vi "运维调试_总磷总氮.vi"() -> ()   [LabVIEW 2016, in "斯坦道总磷总氮.lvlib"]
uses:
  <vilib>/Utility/miscctls.llb/LVPointTypeDef.ctl
  <vilib>/Utility/config.llb/NI_LVConfig.lvlib
  <vilib>/ptbypt/NI_PtbyPt.lvlib
panel:
  out "固件版本号":string
  in  "定时设置":cluster{"启动":bool, "控制命令":T1, "测量参数":T2}(xcontrol)
  out "模块版本号":string
  out "温度2":sgl
  out "温度1":sgl
  out "ADC":sgl
  out "F3":sgl format="%#.6f"
  out "F2":sgl format="%#.6f"
  out "F1":sgl format="%#.6f"
  out "F0":sgl format="%#.6f"
  out "运行状态":T3 {"数据时间:" format="%<%y/%m/%d %H:%M:%S>T"; "仪器时间:" format="%<%y/%m/%d %H:%M:%S>T"}
  in  "单选按钮":enum32{"选项卡 1", "选项卡 2"}(radio)
  in  "总磷参数设置":bool
  in  "总氮参数设置":bool
  out "二级权限":bool
  out "一级权限":bool
  out "输入密码":u32
  out "布尔":bool
  in  "流程固件":bool
  in  "量程参数读取":T4
  in  "模块启用":bool
  in  "串口设置":bool
  in  "公式一键写入":bool
  in  "流程路径":path=path "C:/Users/Hsiao/Documents/斯坦道流程文件/流程.xml"
  in  "曲线模型":cluster{"X^2":dbl, "X":dbl, "B":dbl, "r^2":dbl}(xcontrol)
  out "字符串 2":string
  in  "质控参数设置":bool
  in  "总氮自动测试量程配置":T5
  in  "总磷自动测试量程配置":T5
  in  "数组":string[](array[string])
  in  "量程切换阈值写入":bool
  in  "量程切换阈值读取":bool
  in  "参数下拉列表":enum16{"总磷", "总氮"}(ring)
  in  "量程下拉列表":enum16{"低量程", "高量程"}(ring)
  in  "测量模式下拉列表":enum16{"水样测量", "零点核查", "跨度核查", "标样核查", "加标回收"}(ring)
  in  "公式":cluster{"X^2":dbl, "X":dbl, "b":dbl}
  in  "写公式":bool
  in  "读公式":bool
  in  "返回":bool
  in  "参数设置":bool
  out "集成报警信息":string
  in  "停止":bool
  in  "手动启动":bool
  in  "单步测试":bool
  out "多列列表框":i32(listbox)
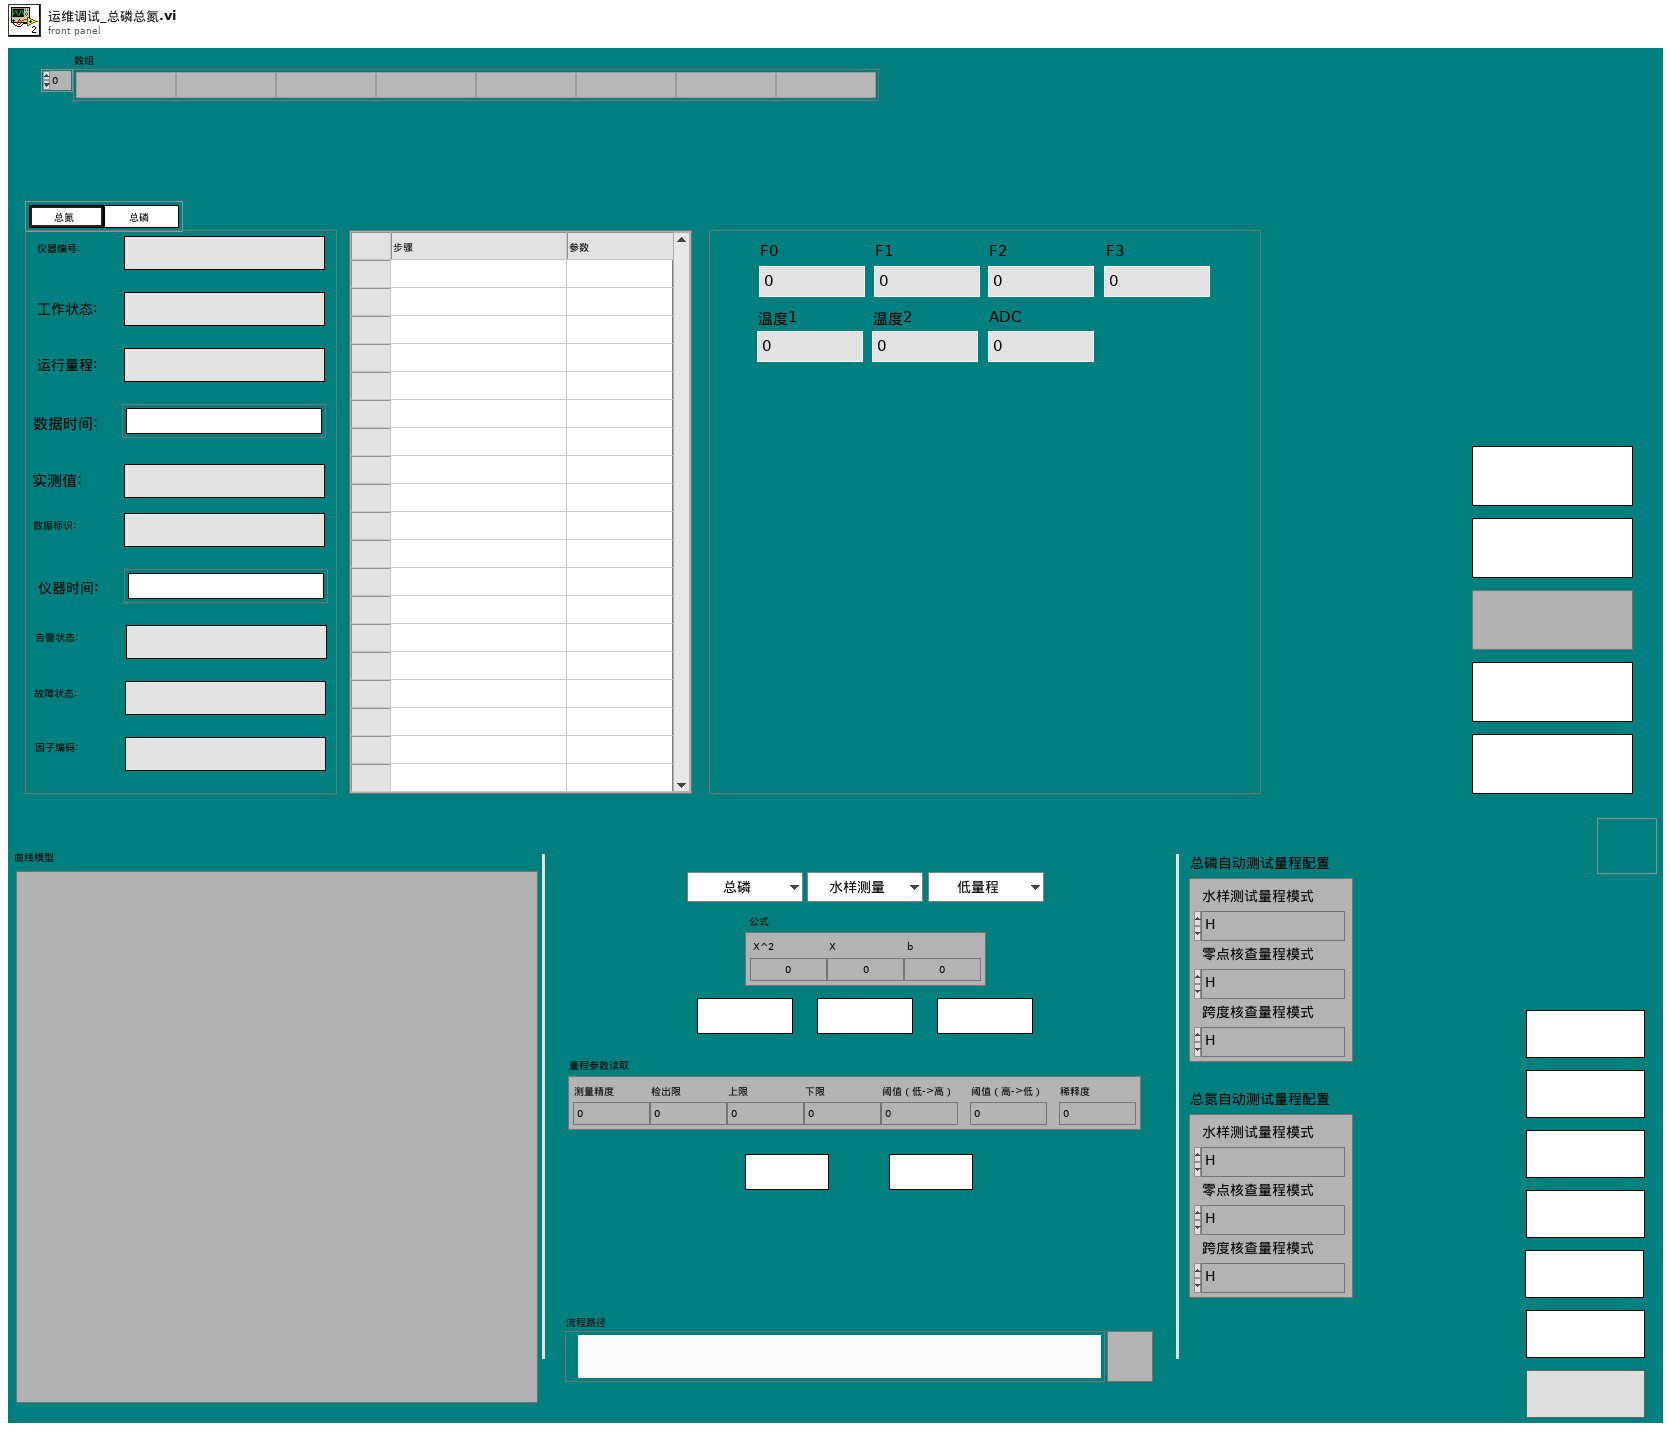
[diagram p1: front panel]
types:
  T1 = typedef "定时设置.xctl/国标控制命令.ctl" = enum16{"启动测量", "标样核查", "零点核查", "跨度核查", "空白测试", "平行样测试", "加标回收", "空白校准", "标样校准", "初始化（清洗）", "停止测试", "仪器重启", "校时", "模式设置", "测量间隔设置"}
  T2 = typedef "定时设置.xctl/测量参数.ctl" = u16
  T3 = cluster{"仪器编号:":string, "工作状态:":string, "运行量程: ":string, "数据时间:":timestamp, "实测值:":string, "数据标识: ":string, "仪器时间:":timestamp, "告警状态: ":string, "故障状态:  ":string, "因子编码:":string}
  T4 = cluster{"测量精度":dbl, "检出限":dbl, "上限":dbl, "下限":dbl, "阈值（低->高）":dbl, "阈值（高->低）":dbl, "稀释度":dbl}
  T5 = cluster{"水样测试量程模式":enum16{"H", "L", "AUTO"}, "空白核查量程模式":enum16{"H", "L", "AUTO"}, "跨度核查量程模式":enum16{"H", "L", "AUTO"}}
  T6 = cluster{"时间源选择":enum16{"系统时间源", "仪器时间源"}, "外部时间源":timestamp}
  T7 = cluster{"系统时间":timestamp, "工作状态":enum16{"空闲", "水样测试", "标样核查", "零点核查", "跨度核查", "空白测试", "平行样测试", "加标回收", "空白校准", "标样校准", "初始化（清洗）"}, "测量模式":enum16{"待机", "连续模式", "周期模式", "定点模式", "受控模式", "手动模式"}, "告警代码":u16, "故障代码":u16, "日志代码":u16, "软件版本":u16, "F0":sgl, "F1":sgl, "F2":sgl, "F3":sgl, "T":sgl, "H":sgl, "id":u16, "flowid":u16, "量程":u16, "总磷控温温度1":sgl, "营养盐控温温度2":sgl, "ADC":sgl}
  T8 = enum16{"空闲", "水样测试", "标样核查", "零点核查", "跨度核查", "空白测试", "平行样测试", "加标回收", "空白校准", "标样校准", "初始化（清洗）"}
  T9 = enum32{"Bad", "Idle", "Run top level", "Running"}
  T10 = typedef "定时设置.xctl/周期模式设置.ctl" = enum16{"不启用", "定点模式", "间隔模式"}
  T11 = typedef "定时设置.xctl/定点周期设置.ctl" = cluster{"启动命令":T12, "启动命令 2":T12, "启动命令 3":T12, "启动命令 4":T12, "启动命令 5":T12, "启动命令 6":T12, "启动命令 7":T12, "启动命令 8":T12, "启动命令 9":T12, "启动命令 10":T12, "启动命令 11":T12, "启动命令 12":T12, "启动命令 13":T12, "启动命令 14":T12, "启动命令 15":T12, "启动命令 16":T12, "启动命令 17":T12, "启动命令 18":T12, "启动命令 19":T12, "启动命令 20":T12, "启动命令 21":T12, "启动命令 22":T12, "启动命令 23":T12, "启动命令 24":T12}
  T12 = typedef "定时设置.xctl/启动命令选择.ctl" = u16
  T13 = typedef "定时设置.xctl/间隔启动设置.ctl" = cluster{"启动命令":T12, "启动间隔":dbl, "启动次数":i32}
  T14 = cluster{"周期模式":T10, "定点周期":T11, "间隔启动":T13, "测量参数":T2}
  T15 = typedef "NI_LVConfig.lvlib/Config Data RefNum.ctl" = refnum<k1>
  T16 = typedef "LVPointTypeDef.ctl" = cluster{"Horizontal":i16, "Vertical":i16}
  T17 = cluster{"因子编码":u32, "单位":u16, "标样参考值":sgl, "水样数据时间":timestamp, "水样实测值":sgl, "水样数据标识":string, "标样数据时间":timestamp, "标样实测值":sgl, "标样数据标识":string, "空白数据时间":timestamp, "空白实测值":sgl, "空白数据标识":string, "零点核查数据时间":timestamp, "零点核查实测值":sgl, "零点核查数据标识":string, "跨度核查数据时间":timestamp, "跨度核查实测值":sgl, "跨度核查数据标识":string, "加标回收数据时间":timestamp, "加标回收实测值":sgl, "加标回收数据标识":string, "平行样数据时间":timestamp, "平行样实测值":sgl, "平行样数据标识":string, "F0":sgl, "F1":sgl, "F2":sgl, "F3":sgl, "F4":sgl, "F5":sgl, "F6":sgl, "F7":sgl, "温度":sgl, "湿度":sgl, "X值":sgl, "fidrange":u16}
  T18 = cluster{"Major":u16, "Minor":u16, "Fix":u16, "Build":u16}
  T19 = enum8{"Enabled", "Disabled", "Disabled and Grayed Out"}
  T20 = cluster{"时间标识":timestamp, "设备":string, "日志信息":string, "备注":string}
  T21 = cluster{"参数":string, "报警内容":string, "报警分析":string}
  T22 = cluster{"启动模式":enum16{"跨度核查", "水样测量", "空白核查", "标样核查", "加标回收"}, "启动参数":u16, "量程":enum16{"低量程", "高量程"}}
  T23 = cluster{"时间标识":timestamp, "设备":string, "日志信息":string, "流程参数":string}
  T24 = typedef "LVRowAndColumnUnsignedTypeDef.ctl" = cluster{"Row":u32, "Column":u32}
  T25 = cluster{"参数下拉列表":enum16{"总磷", "总氮"}, "测量模式下拉列表":enum16{"水样测量", "零点核查", "跨度核查", "标样核查", "加标回收"}, "量程下拉列表":enum16{"低量程", "高量程"}}
  T26 = cluster{"站号":u16, "量程切换":enum32{"H", "L", "AUTO"}, "控制命令":enum16{"启动测量", "标样核查", "零点核查", "跨度核查", "空白测试", "平行样测试", "加标回收", "空白校准", "标样校准", "初始化（清洗）", "停止测试", "仪器重启", "校时", "模式设置", "测量间隔设置"}, "模式设置":enum16{"待机", "连续模式", "周期模式", "定点模式", "受控模式", "手动模式"}, "测量间隔":u16}
  T27 = cluster{"总磷跨度值":dbl, "总磷零点标准液浓度":dbl, "总磷跨度标准液浓度":dbl, "总磷标准液标准浓度":dbl, "总氮跨度值":dbl, "总氮零点标准液浓度":dbl, "总氮跨度标准液浓度":dbl, "总氮标准液标准浓度":dbl}
  T28 = cluster{"确定":bool, "总磷跨度值":dbl, "总磷零点标准液浓度":dbl, "总磷跨度标准液浓度":dbl, "总磷标准液标准浓度":dbl, "总氮跨度值":dbl, "总氮零点标准液浓度":dbl, "总氮跨度标准液浓度":dbl, "总氮标准液标准浓度":dbl}
  T29 = cluster{"测量量程":dbl, "测量精度":dbl, "测量间隔":dbl, "消解温度":dbl, "消解时长":dbl, "空白校准时间":timestamp, "曲线截距":dbl, "曲线斜率":dbl, "测量检出限":dbl, "测量信号值":dbl, "线性相关系数":dbl, "二次多项式系数":dbl, "标样校准时间":timestamp, "稀释倍数":dbl, "三项式系数":dbl, "空白标定系数":dbl, "量程系数":dbl, "F0/ORPA":dbl, "F1/ORPB":dbl, "F2/ORPK":dbl, "F3":dbl, "F4":dbl, "F5":dbl, "F6":dbl, "F7":dbl, "X0/滴定数":dbl, "量程":dbl}
  T30 = cluster{"确定":bool, "测量量程":dbl, "测量精度":dbl, "测量间隔":dbl, "消解温度":dbl, "消解时长":dbl, "空白校准时间":timestamp, "曲线截距":dbl, "曲线斜率":dbl, "测量检出限":dbl, "测量信号值":dbl, "线性相关系数":dbl, "二次多项式系数":dbl, "标样校准时间":timestamp, "稀释倍数":dbl, "三项式系数":dbl, "空白标定系数":dbl, "量程系数":dbl, "F0/ORPA":dbl, "F1/ORPB":dbl, "F2/ORPK":dbl, "F3":dbl, "F4":dbl, "F5":dbl, "F6":dbl, "F7":dbl, "X0/滴定数":dbl, "量程":dbl}
  T31 = cluster{"测量精度":u16, "检出限":dbl, "上限":dbl, "下限":dbl, "阈值（低->高）":dbl, "阈值（高->低）":dbl, "稀释度":dbl}
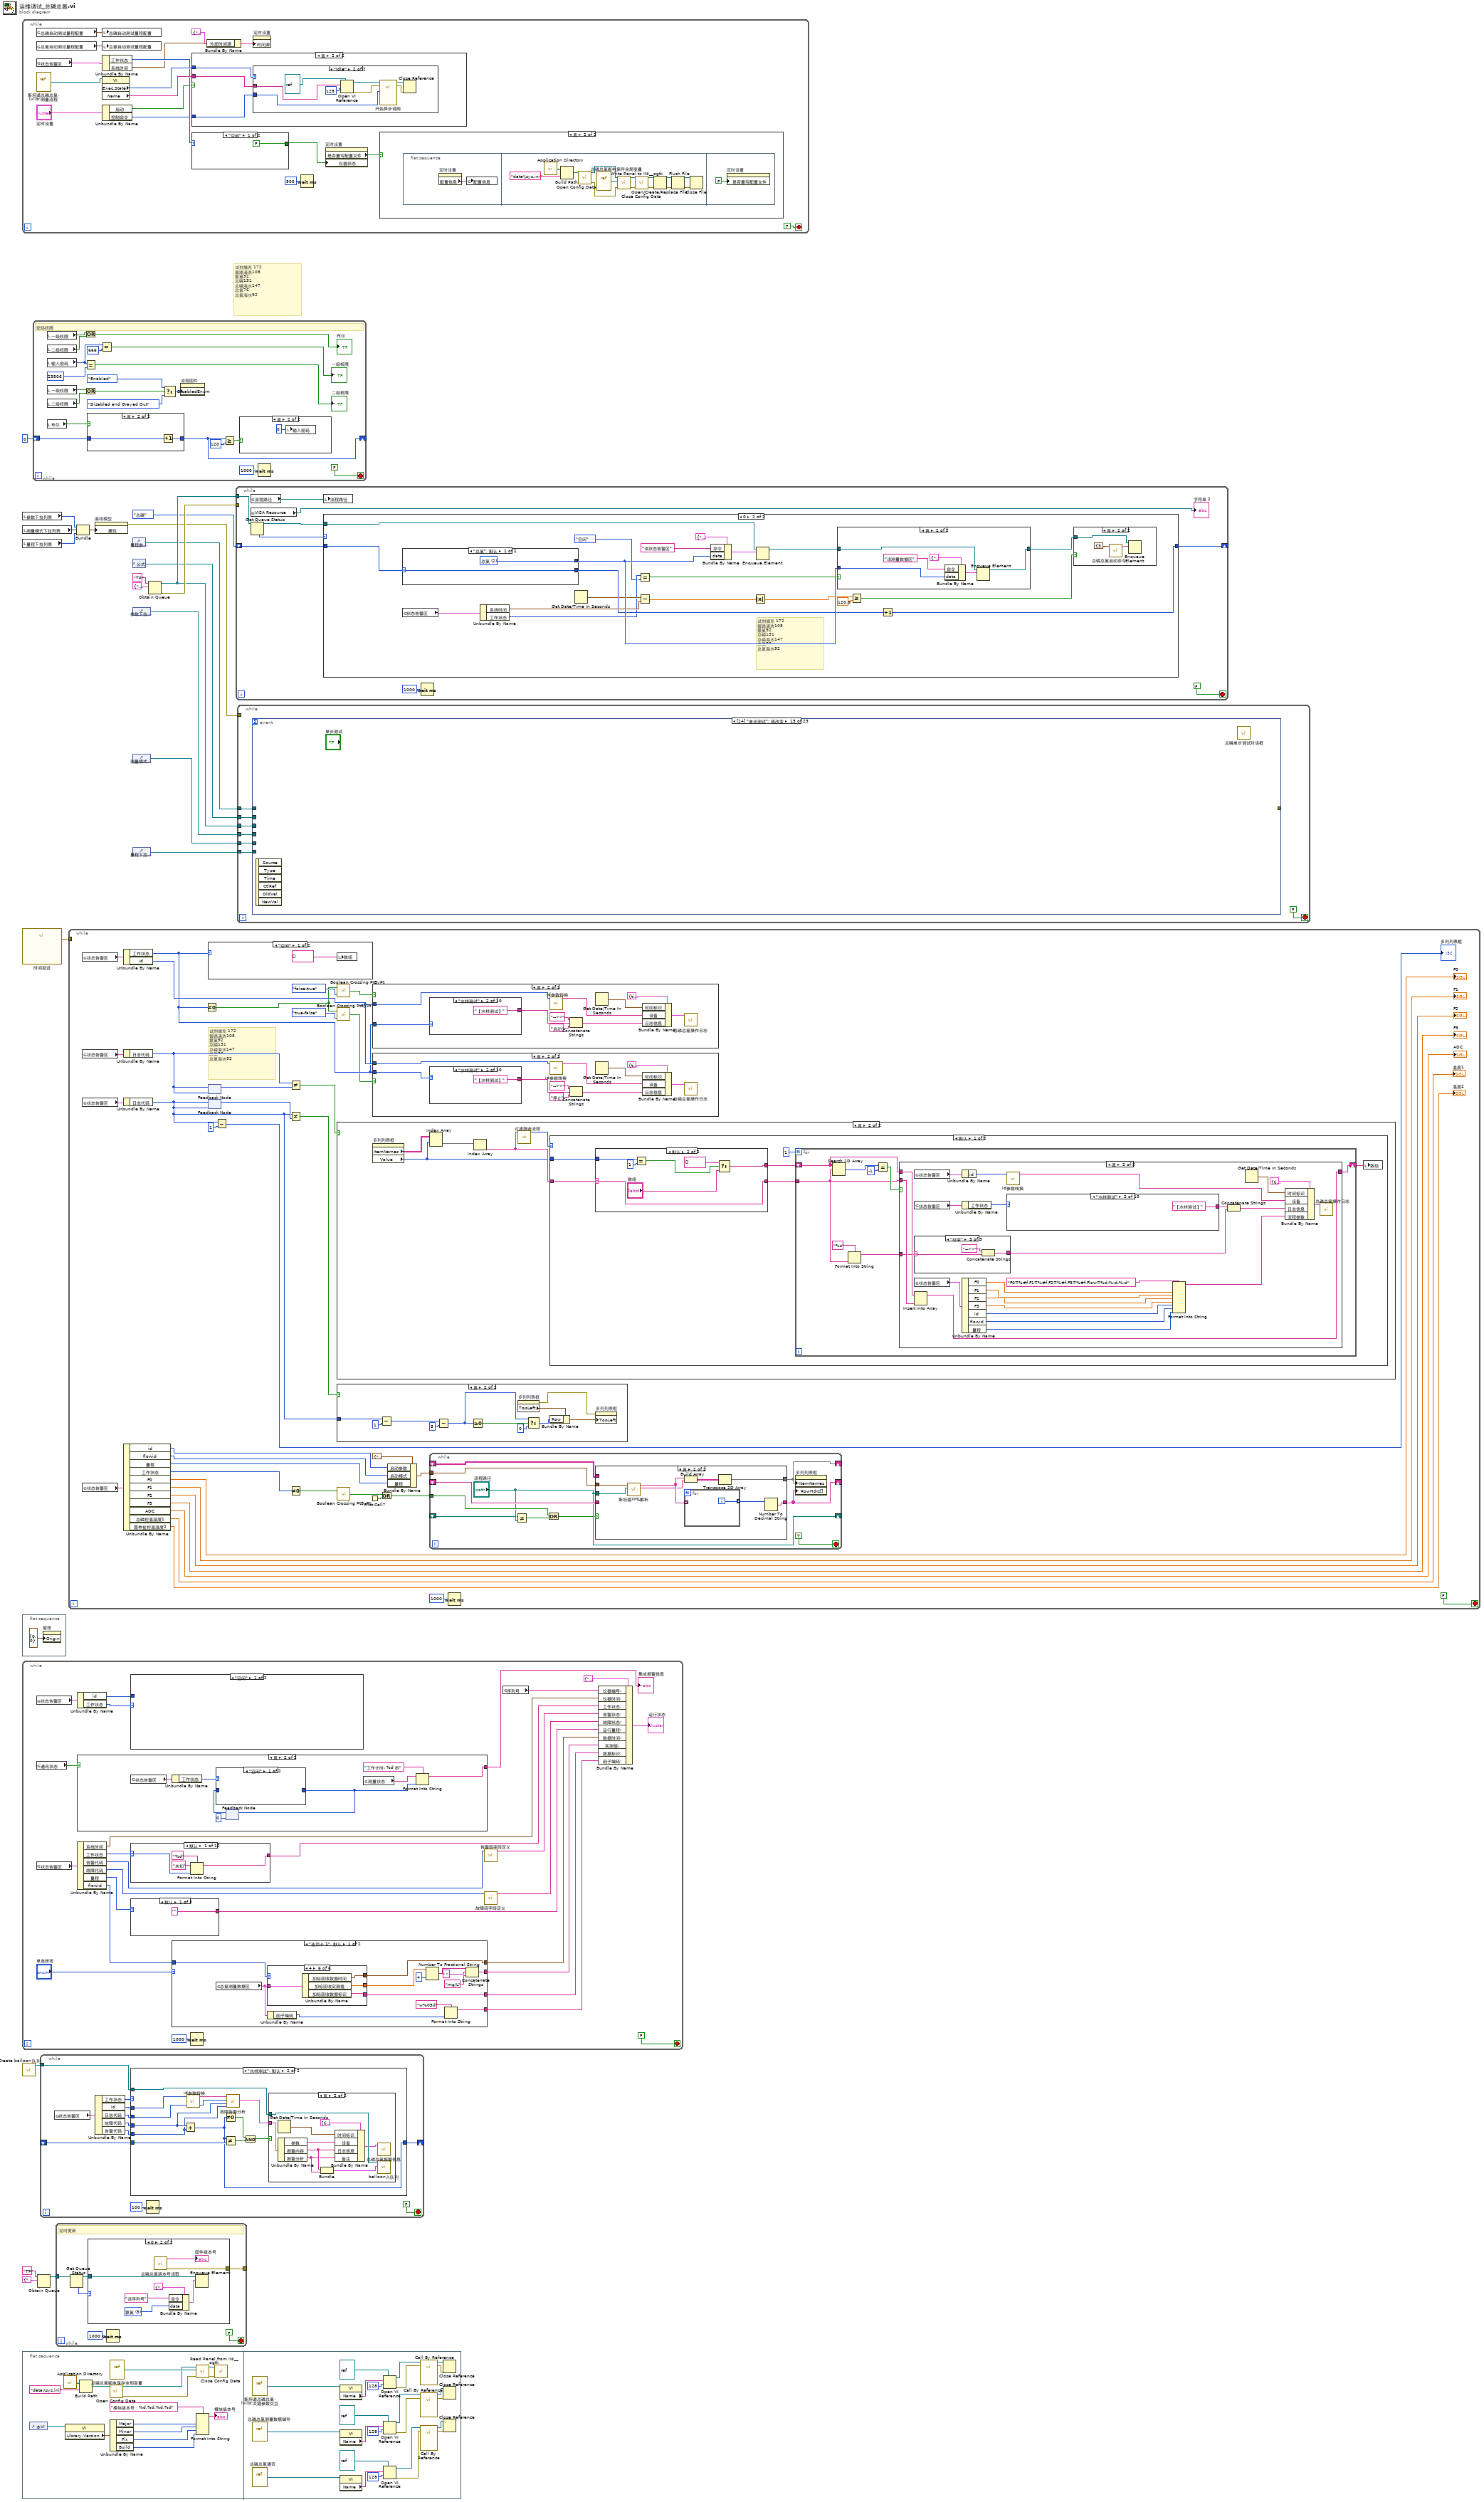
[diagram p0: block diagram]
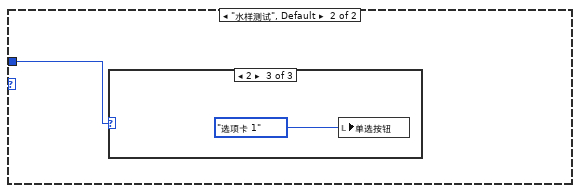
[diagram p7: hidden frame]
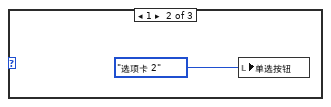
[diagram p9: hidden frame]
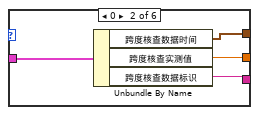
[diagram p11: hidden frame]
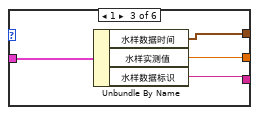
[diagram p12: hidden frame]
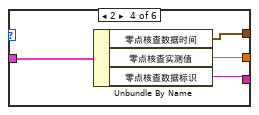
[diagram p13: hidden frame]
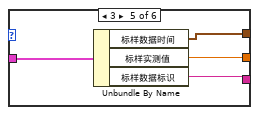
[diagram p14: hidden frame]
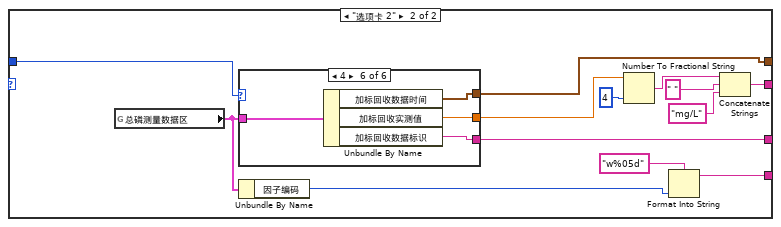
[diagram p15: hidden frame]
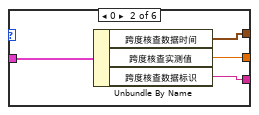
[diagram p17: hidden frame]
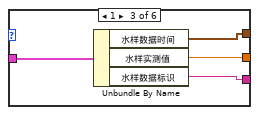
[diagram p18: hidden frame]
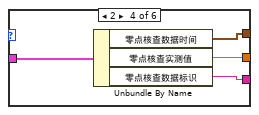
[diagram p19: hidden frame]
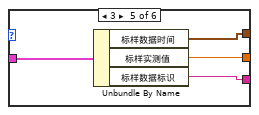
[diagram p20: hidden frame]
diagram:
  # "试剂填充 172 \n管路清洗108\n氨氮92\n总磷131\n总磷海水147\n总氮76\n总氮海水92"
  n1 = while {
    stop <- FALSE stop-if-true
    n2 = global read "总磷总氮断电保存全局变量.vi" "总磷自动测试量程配置"() -> (w35:T5)
    n3 = global read "总磷总氮断电保存全局变量.vi" "总氮自动测试量程配置"() -> (w36:T5)
    n4 = global read "VAR总磷总氮全局变量.vi" "状态告警区"() -> (w31:T7)
    n5 = vi-ref "斯坦道总磷总氮.lvlib:测量流程.vi"() -> (w34:refnum<vi>)
    n6 = local write "总磷自动测试量程配置"(w35) -> ()
    n7 = local write "总氮自动测试量程配置"(w36) -> ()
    n8 = Unbundle By Name(w31) -> ("工作状态"=w30:T8, "系统时间"=w22:timestamp)
    n9 = property class="VI"(reference=w34) -> ("Exec.State"=w33:T9, "Name"=w32:string)  [unwired: 1 in, 2 out]
    n10 = Unbundle By Name("定时设置") -> ("启动"=w26:bool, "控制命令"=w25:T1)
    n11 = case shown="真" w26 {
      tunnel: w32 -> [_ w60]
      tunnel: w25 -> [_ w59]
      tunnel: w33 -> [_ w58]
      frame False {
      }
      frame True {
        n12 = case shown="\"Idle\"" w58 {
          tunnel: w60 -> [_ w64]
          tunnel: w59 -> [_ w61]
          frame "Bad", Default {
          }
          frame "Idle" {
            n13 = Open VI Reference(type specifier VI Refnum (for type only)=refnum<vi> refnum, vi path=w64, options=128 ("选项")) -> (vi reference=w65:refnum<vi>, error out=w66:errorcluster)  [unwired: 3 in]
            n14 = call-by-ref "开始异步调用"(reference=w65, error in=w66, "控制命令"=w61) -> (reference out=w67:refnum<vi>, error out=w68:errorcluster)  [unwired: 11 in]
            n15 = Close Reference(reference=w67, error in (no error)=w68) -> ()  [unwired: 1 out]
          }
        }
      }
    }
    n16 = case shown="\"空闲\"" w30 {
      tunnel: [FALSE TRUE] -> w29
      frame "空闲" {
      }
      frame "水样测试", Default {
      }
    }
    n17 = Bundle By Name(cluster=T6 {"时间源选择"=enum."仪器时间源", "外部时间源"=timestamp(0 s since 1904-01-01)} ("时间源"), "外部时间源"=w22) -> (w23:T6)
    n18 = property on="定时设置" class="定时设置 (严格)"("时间源"=w23) -> ()  [unwired: 2 in, 2 out]
    n19 = Wait (ms)(milliseconds to wait=u32 500 ("等待时间（毫秒）")) -> ()  [unwired: 1 out]
    n20 = property on="定时设置" class="定时设置 (严格)"("仪器状态"=w29) -> ("是否重写配置文件"=w28:bool)  [unwired: 2 in, 2 out]
    n21 = case shown="真" w28 {
      frame False {
        n22 = global read "总磷总氮断电保存全局变量.vi" "配置信息"() -> (w39:T14)
        n23 = property on="定时设置" class="定时设置 (严格)"("配置信息"=w39) -> ()  [unwired: 2 in, 2 out]
      }
      frame True {
        n24 = flat-sequence {
          frame #0 {
            n25 = property on="定时设置" class="定时设置 (严格)"() -> ("配置信息"=w40:T14)  [unwired: 2 in, 2 out]
            n26 = global write "总磷总氮断电保存全局变量.vi" "配置信息"(w40) -> ()
          }
          frame #1 {
            n27 = call <vilib>:"Application Directory.vi"() -> ("Application Directory"=w54:path)
            n28 = Build Path(base path=w54, name or relative path="data\\sys.ini" ("名称或相对路径")) -> (appended path=w52:path)
            n29 = call <vilib>:"Open Config Data.vi"("configuration file path"=w52) -> ("error out"=w48:errorcluster, "refnum"=w51:T15)  [unwired: 8 in, 1 out]
            n30 = vi-ref "总磷总氮断电保存全局变量.vi"() -> (w50:refnum<vi>)
            n31 = call <userlib>:"Write Panel to INI__ogtk.vi"("error in (no error)"=w48, "VI ref"=w50, "refnum"=w51) -> ("error out"=w47:errorcluster, "refnum out"=w49:T15)  [unwired: 7 in]
            n32 = call <vilib>:"Close Config Data.vi"("error in (no error)"=w47, "refnum"=w49) -> ("error out"=w42:errorcluster, "file path"=w41:path)  [unwired: 8 in]
            n33 = Open/Create/Replace File(file path (use dialog)=w41, error in=w42) -> (refnum out=w45:refnum<file>, error out=w46:errorcluster)  [unwired: 4 in, 1 out]
            n34 = Flush File(refnum=w45, error in=w46) -> (refnum out=w44:refnum<file>, error out=w43:errorcluster)
            n35 = Close File(refnum=w44, error in=w43) -> ()  [unwired: 2 out]
          }
          frame #2 {
            n36 = property on="定时设置" class="定时设置 (严格)"("是否重写配置文件"=FALSE) -> ()  [unwired: 2 in, 2 out]
          }
        }
      }
    }
  }
  n37 = local read "参数下拉列表"() -> (w5:enum16{"总磷", "总氮"})
  n38 = local read "测量模式下拉列表"() -> (w4:enum16{"水样测量", "零点核查", "跨度核查", "标样核查", "加标回收"})
  n39 = local read "量程下拉列表"() -> (w3:enum16{"低量程", "高量程"})
  n40 = call "时间延迟"() -> ("error out"=w11:errorcluster)  [unwired: 11 in]
  n41 = flat-sequence {
    frame #0 {
      n42 = property on="窗格" class="Pane"("Origin"=T16 {"Horizontal"=0, "Vertical"=0} ("原点")) -> ()  [unwired: 2 in, 2 out]
    }
  }
  n43 = while {
    stop <- FALSE stop-if-true
    n44 = global read "VAR总磷总氮全局变量.vi" "状态告警区"() -> (w76:T7)
    n45 = global read "VAR总磷总氮全局变量.vi" "通讯状态"() -> (w93:bool)
    n46 = global read "VAR总磷总氮全局变量.vi" "状态告警区"() -> (w91:T7)
    n47 = Unbundle By Name(w76) -> ("id"=w75:u16, "工作状态"=w70:T8)
    n48 = case shown="真" w93 {
      tunnel: ["通讯异常" ("集成报警信息") w185] -> w92
      frame False {
      }
      frame True {
        n49 = global read "VAR总磷总氮全局变量.vi" "状态告警区"() -> (w191:T7)
        n50 = Unbundle By Name(w191) -> ("工作状态"=w190:T8)
        n51 = feedback #1(0) -> (w188:i32)
        n52 = case shown="\"空闲\"" w190 {
          tunnel: w188 -> [_ w193]
          tunnel: [_ w192] -> w186
          frame "空闲" {
          }
          frame Default {
            n53 = Increment(x=w193) -> (x+1=w192:i32)
          }
        }
        n54 = feedback-in #1(w186) -> ()
        n55 = global read "VAR总磷总氮全局变量.vi" "测量状态"() -> (w184:string)
        n56 = Format Into String(format string="工作计时: %d 秒" ("格式字符串"), initial string=w184, w186) -> (resulting string=w185:string)  [unwired: 1 in, 1 out]
      }
    }
    "集成报警信息" <- w92
    n57 = Unbundle By Name(w91) -> ("系统时间"=w87:timestamp, "工作状态"=w86:T8, "告警代码"=w74:u16, "故障代码"=w72:u16, "量程"=w84:u16, "flowid"=w81:u16)
    n58 = case shown="\"空闲\"" w70 {
      tunnel: w75 -> [_ w96]
      frame "空闲" {
      }
      frame "水样测试", Default {
        n59 = case shown="2" w96 {
          frame 0, Default {
          }
          frame 1 {
            n60 = local write "单选按钮"(enum32{"选项卡 1", "选项卡 2"}."选项卡 2" ("单选按钮")) -> ()
          }
          frame 2 {
            n61 = local write "单选按钮"(enum32{"选项卡 1", "选项卡 2"}."选项卡 1" ("单选按钮")) -> ()
          }
        }
      }
    }
    n62 = case shown="默认" w86 {
      selector: w86 -> [w168 _ _ _ _ _ _ _ _ _ _ _]
      tunnel: [w169 "空闲" ("工作状态") "水样测量" ("工作状态") "标样核查" ("工作状态") "零点核查" ("工作状态") "跨度核查" ("工作状态") "空白测试" ("工作状态") "平行样测试" ("工作状态") "加标回收" ("工作状态") "空白校准" ("工作状态") "标样校准" ("工作状态") "初始化" ("工作状态")] -> w85
      frame Default {
        n63 = Format Into String(format string="%d" ("格式字符串"), initial string="未知" ("工作状态"), w168) -> (resulting string=w169:string)  [unwired: 1 in, 1 out]
      }
      frame "空闲" {
      }
      frame "水样测试" {
      }
      frame "标样核查" {
      }
      frame "零点核查" {
      }
      frame "跨度核查" {
      }
      frame "空白测试" {
      }
      frame "平行样测试" {
      }
      frame "加标回收" {
      }
      frame "空白校准" {
      }
      frame "标样校准" {
      }
      frame "初始化（清洗）" {
      }
    }
    n64 = case shown="默认" w84 {
      tunnel: ["" ("字符串") "低量程" ("字符串") "高量程" ("字符串")] -> w83
      frame Default {
      }
      frame 0 {
      }
      frame 1 {
      }
    }
    n65 = case shown="\"选项卡 1\", 默认" "单选按钮" {
      tunnel: w81 -> [w103 w136]
      tunnel: [w102 w135] -> w80
      tunnel: [w101 w134] -> w79
      tunnel: [w100 w133] -> w78
      tunnel: [w99 w132] -> w77
      frame "选项卡 1", Default {
        n66 = global read "VAR总磷总氮全局变量.vi" "总氮测量数据区"() -> (w104:T17)
        n67 = case shown="4" w103 {
          tunnel: [_ w115 w119 w123 w127 w131] -> w102
          tunnel: [_ w113 w118 w122 w126 w130] -> w106
          tunnel: [_ w112 w117 w121 w125 w129] -> w100
          tunnel: w104 -> [_ w114 w116 w120 w124 w128]
          frame Default {
          }
          frame 0 {
            n68 = Unbundle By Name(w114) -> ("跨度核查数据时间"=w115:timestamp, "跨度核查实测值"=w113:sgl, "跨度核查数据标识"=w112:string)
          }
          frame 1 {
            n69 = Unbundle By Name(w116) -> ("水样数据时间"=w119:timestamp, "水样实测值"=w118:sgl, "水样数据标识"=w117:string)
          }
          frame 2 {
            n70 = Unbundle By Name(w120) -> ("零点核查数据时间"=w123:timestamp, "零点核查实测值"=w122:sgl, "零点核查数据标识"=w121:string)
          }
          frame 3 {
            n71 = Unbundle By Name(w124) -> ("标样数据时间"=w127:timestamp, "标样实测值"=w126:sgl, "标样数据标识"=w125:string)
          }
          frame 4 {
            n72 = Unbundle By Name(w128) -> ("加标回收数据时间"=w131:timestamp, "加标回收实测值"=w130:sgl, "加标回收数据标识"=w129:string)
          }
        }
        n73 = Unbundle By Name(w104) -> ("因子编码"=w110:u32)
        n74 = Number To Fractional String(number=w106, precision (6)=i16 4 ("精度(6)")) -> (F-format string=w108:string)  [unwired: 2 in]
        n75 = Format Into String(format string="w%05d" ("格式字符串"), w110) -> (resulting string=w99:string)  [unwired: 2 in, 1 out]
        n76 = Concatenate Strings(w108, " " ("字符串"), "mg/L" ("字符串")) -> (w101:string)
      }
      frame "选项卡 2" {
        n77 = global read "VAR总磷总氮全局变量.vi" "总磷测量数据区"() -> (w137:T17)
        n78 = case shown="4" w136 {
          tunnel: [_ w148 w152 w156 w160 w164] -> w135
          tunnel: [_ w146 w151 w155 w159 w163] -> w139
          tunnel: [_ w145 w150 w154 w158 w162] -> w133
          tunnel: w137 -> [_ w147 w149 w153 w157 w161]
          frame Default {
          }
          frame 0 {
            n79 = Unbundle By Name(w147) -> ("跨度核查数据时间"=w148:timestamp, "跨度核查实测值"=w146:sgl, "跨度核查数据标识"=w145:string)
          }
          frame 1 {
            n80 = Unbundle By Name(w149) -> ("水样数据时间"=w152:timestamp, "水样实测值"=w151:sgl, "水样数据标识"=w150:string)
          }
          frame 2 {
            n81 = Unbundle By Name(w153) -> ("零点核查数据时间"=w156:timestamp, "零点核查实测值"=w155:sgl, "零点核查数据标识"=w154:string)
          }
          frame 3 {
            n82 = Unbundle By Name(w157) -> ("标样数据时间"=w160:timestamp, "标样实测值"=w159:sgl, "标样数据标识"=w158:string)
          }
          frame 4 {
            n83 = Unbundle By Name(w161) -> ("加标回收数据时间"=w164:timestamp, "加标回收实测值"=w163:sgl, "加标回收数据标识"=w162:string)
          }
        }
        n84 = Unbundle By Name(w137) -> ("因子编码"=w143:u32)
        n85 = Number To Fractional String(number=w139, precision (6)=i16 4 ("精度(6)")) -> (F-format string=w141:string)  [unwired: 2 in]
        n86 = Format Into String(format string="w%05d" ("格式字符串"), w143) -> (resulting string=w132:string)  [unwired: 2 in, 1 out]
        n87 = Concatenate Strings(w141, " " ("字符串"), "mg/L" ("字符串")) -> (w134:string)
      }
    }
    n88 = Wait (ms)(milliseconds to wait=u32 1000 ("等待时间（毫秒）")) -> ()  [unwired: 1 out]
    n89 = call "告警码字段定义.vi"("告警代码"=w74) -> ("字符串"=w73:string)  [unwired: 8 in, 2 out]
    n90 = call "故障码字段定义.vi"("故障代码"=w72) -> ("字符串"=w71:string)  [unwired: 10 in]
    n91 = global read "VAR总磷总氮全局变量.vi" "序列号"() -> (w88:string)
    n92 = Bundle By Name(cluster=T3 {"仪器编号:"="", "工作状态:"="", "运行量程: "="", "数据时间:"=timestamp(0 s since 1904-01-01), "实测值:"="", "数据标识: "="", "仪器时间:"=timestamp(0 s since 1904-01-01), "告警状态: "="", "故障状态:  "="", "因子编码:"=""} ("运行状态"), "仪器编号:"=w88, "仪器时间:"=w87, "工作状态:"=w85, "告警状态:"=w73, "故障状态:"=w71, "运行量程:"=w83, "数据时间:"=w80, "实测值:"=w79, "数据标识:"=w78, "因子编码:"=w77) -> (→"运行状态":T3)
  }
  n93 = call "Create balloon 队列.vi"() -> ("队列输出"=w1:refnum<queue>)  [unwired: 11 in]
  n94 = flat-sequence {
    frame #0 {
      n95 = control-ref of="本VI"() -> (w201:refnum<vi>)
      n96 = call <vilib>:"Application Directory.vi"() -> ("Application Directory"=w202:path)
      n97 = property class="VI"(reference=w201) -> ("Library.Version"=w200:T18)  [unwired: 1 in, 2 out]
      n98 = Build Path(base path=w202, name or relative path="data\\sys.ini" ("名称或相对路径")) -> (appended path=w204:path)
      n99 = vi-ref "总磷总氮断电保存全局变量.vi"() -> (w206:refnum<vi>)
      n100 = call <vilib>:"Open Config Data.vi"("configuration file path"=w204) -> ("error out"=w208:errorcluster, "refnum"=w205:T15)  [unwired: 8 in, 1 out]
      n101 = Unbundle By Name(w200) -> ("Major"=w198:u16, "Minor"=w197:u16, "Fix"=w196:u16, "Build"=w195:u16)
      n102 = call <userlib>:"Read Panel from INI__ogtk.vi"("error in (no error)"=w208, "VI ref"=w206, "refnum"=w205) -> ("error out"=w209:errorcluster, "refnum out"=w207:T15)  [unwired: 7 in]
      n103 = Format Into String(format string="模块版本号：%d.%d.%d.%d" ("格式字符串"), w198, w197, w196, w195) -> (resulting string=→"模块版本号":string)  [unwired: 2 in, 1 out]
      n104 = call <vilib>:"Close Config Data.vi"("error in (no error)"=w209, "refnum"=w207) -> ()  [unwired: 8 in, 2 out]
    }
    frame #1 {
      n105 = vi-ref "斯坦道总磷总氮.lvlib:关键参数交互.vi"() -> (w217:refnum<vi>)
      n106 = vi-ref "总磷总氮测量数据储存.vi"() -> (w226:refnum<vi>)
      n107 = vi-ref "总磷总氮通讯.vi"() -> (w218:refnum<vi>)
      n108 = property class="VI"(reference=w217) -> ("Name"=w211:string)  [unwired: 1 in, 2 out]
      n109 = property class="VI"(reference=w226) -> ("Name"=w233:string)  [unwired: 1 in, 2 out]
      n110 = property class="VI"(reference=w218) -> ("Name"=w219:string)  [unwired: 1 in, 2 out]
      n111 = Open VI Reference(type specifier VI Refnum (for type only)=refnum<vi> refnum, vi path=w211, options=128 ("选项")) -> (vi reference=w213:refnum<vi>, error out=w214:errorcluster)  [unwired: 3 in]
      n112 = Open VI Reference(type specifier VI Refnum (for type only)=refnum<vi> refnum, vi path=w233, options=128 ("选项")) -> (vi reference=w231:refnum<vi>, error out=w229:errorcluster)  [unwired: 3 in]
      n113 = Open VI Reference(type specifier VI Refnum (for type only)=refnum<vi> refnum, vi path=w219, options=128 ("选项")) -> (vi reference=w221:refnum<vi>, error out=w223:errorcluster)  [unwired: 3 in]
      n114 = call-by-ref "?"(reference=w213, error in=w214) -> (reference out=w216:refnum<vi>, error out=w215:errorcluster)  [unwired: 12 in]
      n115 = call-by-ref "?"(reference=w231, error in=w229) -> (reference out=w227:refnum<vi>, error out=w228:errorcluster)  [unwired: 12 in]
      n116 = call-by-ref "?"(reference=w221, error in=w223) -> (reference out=w225:refnum<vi>, error out=w224:errorcluster)  [unwired: 12 in]
      n117 = Close Reference(reference=w216, error in (no error)=w215) -> ()  [unwired: 1 out]
      n118 = Close Reference(reference=w227, error in (no error)=w228) -> ()  [unwired: 1 out]
      n119 = Close Reference(reference=w225, error in (no error)=w224) -> ()  [unwired: 1 out]
    }
  }
  n120 = while {
    shift-right: [w242] -> _
    shift-left: u32 0 ("y") -> [w244]
    stop <- FALSE stop-if-true
    # "密码权限"
    n121 = local read "一级权限"() -> (w247:bool)
    n122 = local read "二级权限"() -> (w248:bool)
    n123 = local read "输入密码"() -> (w251:u32)
    n124 = local read "一级权限"() -> (w238:bool)
    n125 = local read "二级权限"() -> (w239:bool)
    n126 = local read "布尔"() -> (w245:bool)
    n127 = Or(x=w247, y=w248) -> (x .or. y?=→"布尔":bool)
    n128 = Equal?(x=w251, y=u32 23506) -> (x = y?=→"二级权限":bool)
    n129 = Or(x=w238, y=w239) -> (x .or. y?=w237:bool)
    n130 = case shown="真" w245 {
      tunnel: w244 -> [_ w257]
      tunnel: [_ w256] -> w242
      frame False {
      }
      frame True {
        n131 = Increment(x=w257) -> (x+1=w256:u32)
      }
    }
    n132 = Equal?(x=w251, y=u32 666) -> (x = y?=→"一级权限":bool)
    n133 = Select(t=T19."Enabled" ("禁用"), s=w237, f=T19."Disabled and Grayed Out" ("禁用")) -> (s? t:f=w234:T19)
    n134 = property on="流程固件" class="Bool"("DisabledEnum"=w234) -> ()  [unwired: 2 in, 2 out]
    n135 = Greater Or Equal?(x=w242, y=u32 120) -> (x >= y?=w240:bool)
    n136 = case shown="真" w240 {
      frame False {
      }
      frame True {
        n137 = local write "输入密码"(u32 0 ("输入密码")) -> ()
      }
    }
    n138 = Wait (ms)(milliseconds to wait=u32 1000 ("等待时间（毫秒）")) -> ()  [unwired: 1 out]
  }
  n139 = Obtain Queue(name (unnamed)="TP" ("名称（未命名）"), element data type=cluster{"命令":string, "data":variant} {"命令"="", "data"=variant}) -> (queue out=w8:refnum<queue>)  [unwired: 3 in, 2 out]
  n140 = while {
    tunnel: w1 -> [w264]
    shift-right: [w260] -> _
    shift-left: _ -> [w261]
    stop <- FALSE stop-if-true
    n141 = global read "VAR总磷总氮全局变量.vi" "状态告警区"() -> (w258:T7)
    n142 = Unbundle By Name(w258) -> ("工作状态"=w259:T8, "id"=w266:u16, "日志代码"=w265:u16, "故障代码"=w263:u16, "告警代码"=w262:u16)
    n143 = case shown="\"水样测试\", 默认" w259 {
      tunnel: w266 -> [_ w281]
      tunnel: w265 -> [_ w280]
      tunnel: w264 -> [_ w277]
      tunnel: w263 -> [_ w276]
      tunnel: w262 -> [_ w275]
      tunnel: w261 -> [w269 w274]
      tunnel: [w269 w273] -> w260
      frame "空闲" {
      }
      frame "水样测试", Default {
        n144 = Add(x=w276, y=w275) -> (x+y=w273:u16)
        n145 = call "id参数转换.vi"("id"=w281) -> ("table输出"=w278:string)  [unwired: 10 in]
        n146 = Not Equal To 0?(x=w273) -> (x != 0?=w272:bool)
        n147 = Not Equal?(x=w273, y=w274) -> (x != y?=w271:bool)
        n148 = call "故障告警分析.vi"("告警代码"=w275, "故障代码"=w276, "运行步序"=w280, "参数"=w278) -> ("报警内容"=w279:T21)  [unwired: 6 in, 1 out]
        n149 = And(x=w272, y=w271) -> (x .and. y?=w270:bool)
        n150 = case shown="真" w270 {
          tunnel: w279 -> [_ w290]
          tunnel: w277 -> [_ w289]
          frame False {
          }
          frame True {
            n151 = Get Date/Time In Seconds() -> (seconds since 1Jan1904=w288:timestamp)
            n152 = Unbundle By Name(w290) -> ("参数"=w285:string, "报警内容"=w284:string, "报警分析"=w283:string)
            n153 = Bundle("报警内容"=w284, "报警分析"=w283) -> (w282:cluster{"报警内容":string, "报警分析":string})  [unwired: 1 in]
            n154 = Bundle By Name(cluster=T20 {"时间标识"=timestamp(0 s since 1904-01-01), "设备"="", "日志信息"="", "备注"=""} ("data in"), "时间标识"=w288, "设备"=w285, "日志信息"=w284, "备注"=w283) -> (w287:T20)
            n155 = call "总磷总氮报警信息.vi"("data in"=w287) -> ()  [unwired: 10 in, 1 out]
            n156 = call "balloon入队列.vi"("报警内容"=w282, "队列"=w289) -> ()  [unwired: 9 in, 1 out]
          }
        }
      }
    }
    n157 = Wait (ms)(milliseconds to wait=u32 100) -> ()  [unwired: 1 out]
  }
  n158 = while {
    tunnel: w8 -> [w295]
    tunnel: [w293] -> _
    stop <- FALSE stop-if-true
    # "定时更新"
    n159 = Get Queue Status(queue=w295) -> (queue out=w292:refnum<queue>, # elements in queue=w291:i32)  [unwired: 2 in, 6 out]
    n160 = case shown="0" w291 {
      tunnel: w292 -> [_ w300]
      tunnel: [_ w298] -> w293
      frame Default {
      }
      frame 0 {
        w301 = u16 3 items=["总磷"=1, "氨氮"=3] ("站号")
        n161 = call "总磷总氮版本号读取.vi"() -> ("error out"=w298:errorcluster, "固件版本号"=→"固件版本号":string)  [unwired: 10 in]
        n162 = Bundle By Name(cluster=cluster{"命令":string, "data":variant} {"命令"="", "data"=variant} ("元素"), "命令"="读序列号", "data"=w301) -> (w299:cluster{"命令":string, "data":variant})
        n163 = Enqueue Element(queue=w300, element=w299) -> ()  [unwired: 2 in, 3 out]
      }
    }
    n164 = Wait (ms)(milliseconds to wait=u32 1000 ("等待时间（毫秒）")) -> ()  [unwired: 1 out]
  }
  n165 = while {
    tunnel: w11 -> [_]
    stop <- FALSE stop-if-true
    # "试剂填充 172 \n管路清洗108\n氨氮92\n总磷131\n总磷海水147\n总氮76\n总氮海水92"
    n166 = global read "VAR总磷总氮全局变量.vi" "状态告警区"() -> (w328:T7)
    n167 = global read "VAR总磷总氮全局变量.vi" "状态告警区"() -> (w326:T7)
    n168 = global read "VAR总磷总氮全局变量.vi" "状态告警区"() -> (w330:T7)
    n169 = global read "VAR总磷总氮全局变量.vi" "状态告警区"() -> (w334:T7)
    n170 = Unbundle By Name(w328) -> ("工作状态"=w314:T8, "id"=w315:u16)
    n171 = Unbundle By Name(w326) -> ("日志代码"=w325:u16)
    n172 = Unbundle By Name(w330) -> ("日志代码"=w322:u16)
    n173 = Unbundle By Name(w334) -> ("id"=w331:u16, "flowid"=w333:u16, "量程"=w332:u16, "工作状态"=w319:T8, "F0"=→"F0":sgl, "F1"=→"F1":sgl, "F2"=→"F2":sgl, "F3"=→"F3":sgl, "ADC"=→"ADC":sgl, "总磷控温温度1"=→"温度1":sgl, "营养盐控温温度2"=→"温度2":sgl)
    n174 = Not Equal To 0?(x=w314) -> (x != 0?=w312:bool)
    n175 = case shown="\"空闲\"" w314 {
      frame "空闲" {
        n176 = local write "数组"(string[] [] ("数组")) -> ()
      }
      frame "水样测试", Default {
      }
    }
    n177 = feedback #2(w325) -> (w327:u16)
    n178 = feedback-in #2(w325) -> ()
    n179 = feedback-in #3(w322) -> ()
    n180 = feedback #3(w322) -> (w339:u16)
    n181 = Subtract(x=w322, y=1) -> (x-y=→"多列列表框":i32)
    n182 = Not Equal?(x=w325, y=w327) -> (x != y?=w324:bool)
    n183 = Not Equal?(x=w322, y=w339) -> (x != y?=w338:bool)
    n184 = Not Equal To 0?(x=w319) -> (x != 0?=w336:bool)
    n185 = call <vilib>:"Boolean Crossing PtByPt.vi"("direction"=enum16{"either", "false-true", "true-false"}."false-true", "input"=w312) -> ("crossing"=w316:bool)  [unwired: 1 in]
    n186 = call <vilib>:"Boolean Crossing PtByPt.vi"("direction"=enum16{"either", "false-true", "true-false"}."true-false", "input"=w312) -> ("crossing"=w311:bool)  [unwired: 1 in]
    n187 = case shown="真" w324 {
      frame False {
      }
      frame True {
        n188 = property on="多列列表框" class="MCListbox (严格)"() -> ("ItemNames"=w385:string[][], "Value"=w381:i32)  [unwired: 2 in, 2 out]
        n189 = Index Array(array=w385, index (row)=w381) -> (element=w384:string[])  [unwired: 1 in]
        n190 = Index Array(array=w384) -> (element=w383:string)  [unwired: 1 in]
        n191 = call "过滤筛选流程.vi"("字符串"=w383) -> ("匹配后偏移量"=w382:i32)  [unwired: 10 in]
        n192 = case shown="默认" w382 {
          tunnel: w383 -> [w387 _]
          tunnel: w381 -> [w386 _]
          frame Default {
            n193 = case shown="默认" w387 {
              selector: w387 -> [w393 w400]
              tunnel: [w393 w400] -> w389
              tunnel: [string[] [] ("数组") w395] -> w388
              tunnel: w386 -> [_ w399]
              frame "读数" {
              }
              frame Default {
                n194 = Equal?(x=w399, y=1) -> (x = y?=w397:bool)
                n195 = Select(t=string[] [], s=w397, f="数组") -> (s? t:f=w395:string[])
              }
            }
            n196 = for {
              N: 1 -> [_]
              tunnel: w389 -> [w402]
              shift-right: [w401] -> w390
              shift-left: w388 -> [w403]
              n197 = Search 1D Array(1D array=w403, element=w402) -> (index of element=w406:i32)  [unwired: 1 in]
              n198 = Format Into String(format string="%s" ("格式字符串"), w402) -> (resulting string=w407:string)  [unwired: 2 in, 1 out]
              n199 = Equal?(x=w406, y=-1) -> (x = y?=w404:bool)
              n200 = case shown="真" w404 {
                tunnel: w407 -> [_ w417]
                tunnel: w403 -> [w409 w421]
                tunnel: w402 -> [_ w420]
                tunnel: [w409 w419] -> w401
                frame False {
                }
                frame True {
                  n201 = global read "VAR总磷总氮全局变量.vi" "状态告警区"() -> (w434:T7)
                  n202 = global read "VAR总磷总氮全局变量.vi" "状态告警区"() -> (w415:T7)
                  n203 = case shown="\"结束\"" w417 {
                    selector: w417 -> [w444 w447 w450]
                    tunnel: [w444 w446 w449] -> w416
                    frame Default {
                    }
                    frame "初始化" {
                      n204 = Concatenate Strings("-->>" ("字符串"), w447) -> (w446:string)
                    }
                    frame "结束" {
                      n205 = Concatenate Strings("-->>" ("字符串"), w450) -> (w449:string)
                    }
                  }
                  n206 = global read "VAR总磷总氮全局变量.vi" "状态告警区"() -> (w431:T7)
                  n207 = Insert Into Array(array=w421, new element=w420) -> (w419:string[])  [unwired: 1 in]
                  n208 = Unbundle By Name(w434) -> ("id"=w411:u16)
                  n209 = Unbundle By Name(w415) -> ("工作状态"=w414:T8)
                  n210 = Unbundle By Name(w431) -> ("F0"=w428:sgl, "F1"=w427:sgl, "F2"=w426:sgl, "F3"=w425:sgl, "id"=w424:u16, "flowid"=w423:u16, "量程"=w422:u16)
                  n211 = call "id参数转换.vi"("id"=w411) -> ("table输出"=w410:string)  [unwired: 10 in]
                  n212 = case shown="\"水样测试\"" w414 {
                    tunnel: [_ "【水样测试】" ("字符串") "【标样核查】" ("字符串") "【零点核查】" ("字符串") "【跨度核查】" ("字符串") "【空白测试】" ("字符串") "【平行样测试】" ("字符串") "【加标回收】" ("字符串") "【空白校准】" ("字符串") "【标样校准】" ("字符串")] -> w412
                    frame "空闲", Default {
                    }
                    frame "水样测试" {
                    }
                    frame "标样核查" {
                    }
                    frame "零点核查" {
                    }
                    frame "跨度核查" {
                    }
                    frame "空白测试" {
                    }
                    frame "平行样测试" {
                    }
                    frame "加标回收" {
                    }
                    frame "空白校准" {
                    }
                    frame "标样校准" {
                    }
                  }
                  n213 = Format Into String(format string="F0=%#f,F1=%#f,F2=%#f,F3=%#f,Flow=%d-%-d-%-d" ("格式字符串"), w428, w427, w426, w425, w424, w423, w422) -> (resulting string=w429:string)  [unwired: 2 in, 1 out]
                  n214 = Concatenate Strings(w412, w416) -> (w413:string)
                  n215 = Get Date/Time In Seconds() -> (seconds since 1Jan1904=w432:timestamp)
                  n216 = Bundle By Name(cluster=T23 {"时间标识"=timestamp(0 s since 1904-01-01), "设备"="", "日志信息"="", "流程参数"=""} ("data in"), "时间标识"=w432, "设备"=w410, "日志信息"=w413, "流程参数"=w429) -> (w433:T23)
                  n217 = call "总磷总氮操作日志.vi"("data in"=w433) -> ()  [unwired: 11 in]
                }
              }
            }
            n218 = local write "数组"(w390) -> ()
          }
          frame -1 {
          }
        }
      }
    }
    n219 = case shown="真" w338 {
      tunnel: w322 -> [_ w475]
      frame False {
      }
      frame True {
        n220 = Subtract(x=w475, y=1) -> (x-y=w473:i32)
        n221 = Subtract(x=w473, y=5) -> (x-y=w477:i32)
        n222 = Greater Or Equal To 0?(x=w477) -> (x >= 0?=w476:bool)
        n223 = property on="多列列表框" class="MCListbox (严格)"() -> (error out=w481:errorcluster, "TopLeft"=w482:T24)  [unwired: 2 in, 1 out]
        n224 = Select(t=w477, s=w476, f=0) -> (s? t:f=w478:i32)
        n225 = Bundle By Name(cluster=w482, "Row"=w478) -> (w483:T24)
        n226 = property on="多列列表框" class="MCListbox (严格)"(error in=w481, "TopLeft"=w483) -> ()  [unwired: 1 in, 2 out]
      }
    }
    n227 = call <vilib>:"Boolean Crossing PtByPt.vi"("input"=w336) -> ("crossing"=w318:bool)  [unwired: 2 in]
    n228 = First Call?() -> (First Call?: T/F=w337:bool)
    n229 = case shown="真" w316 {
      tunnel: w314 -> [_ w365]
      tunnel: w315 -> [_ w362]
      frame False {
      }
      frame True {
        n230 = case shown="\"水样测试\"" w365 {
          tunnel: [_ "【水样测试】" ("字符串") "【标样核查】" ("字符串") "【零点核查】" ("字符串") "【跨度核查】" ("字符串") "【空白测试】" ("字符串") "【平行样测试】" ("字符串") "【加标回收】" ("字符串") "【空白校准】" ("字符串") "【标样校准】" ("字符串")] -> w370
          frame "空闲", Default {
          }
          frame "水样测试" {
          }
          frame "标样核查" {
          }
          frame "零点核查" {
          }
          frame "跨度核查" {
          }
          frame "空白测试" {
          }
          frame "平行样测试" {
          }
          frame "加标回收" {
          }
          frame "空白校准" {
          }
          frame "标样校准" {
          }
        }
        n231 = call "id参数转换.vi"("id"=w362) -> ("table输出"=w361:string)  [unwired: 10 in]
        n232 = Concatenate Strings("-->>" ("字符串"), w370, "启动" ("字符串")) -> (w369:string)
        n233 = Get Date/Time In Seconds() -> (seconds since 1Jan1904=w367:timestamp)
        n234 = Bundle By Name(cluster=T23 {"时间标识"=timestamp(0 s since 1904-01-01), "设备"="", "日志信息"="", "流程参数"=""} ("data in"), "时间标识"=w367, "设备"=w361, "日志信息"=w369) -> (w366:T23)
        n235 = call "总磷总氮操作日志.vi"("data in"=w366) -> ()  [unwired: 11 in]
      }
    }
    n236 = case shown="真" w311 {
      tunnel: w314 -> [_ w346]
      tunnel: w315 -> [_ w343]
      frame False {
      }
      frame True {
        n237 = case shown="\"水样测试\"" w346 {
          tunnel: [_ "【水样测试】" ("字符串") "【标样核查】" ("字符串") "【零点核查】" ("字符串") "【跨度核查】" ("字符串") "【空白测试】" ("字符串") "【平行样测试】" ("字符串") "【加标回收】" ("字符串") "【空白校准】" ("字符串") "【标样校准】" ("字符串")] -> w351
          frame "空闲", Default {
          }
          frame "水样测试" {
          }
          frame "标样核查" {
          }
          frame "零点核查" {
          }
          frame "跨度核查" {
          }
          frame "空白测试" {
          }
          frame "平行样测试" {
          }
          frame "加标回收" {
          }
          frame "空白校准" {
          }
          frame "标样校准" {
          }
        }
        n238 = call "id参数转换.vi"("id"=w343) -> ("table输出"=w342:string)  [unwired: 10 in]
        n239 = Concatenate Strings("-->>" ("字符串"), w351, "停止" ("字符串")) -> (w350:string)
        n240 = Get Date/Time In Seconds() -> (seconds since 1Jan1904=w348:timestamp)
        n241 = Bundle By Name(cluster=T23 {"时间标识"=timestamp(0 s since 1904-01-01), "设备"="", "日志信息"="", "流程参数"=""} ("data in"), "时间标识"=w348, "设备"=w342, "日志信息"=w350) -> (w347:T23)
        n242 = call "总磷总氮操作日志.vi"("data in"=w347) -> ()  [unwired: 11 in]
      }
    }
    n243 = Or(x=w318, y=w337) -> (x .or. y?=w335:bool)
    n244 = Bundle By Name(cluster=T22 {"启动模式"=enum."跨度核查", "启动参数"=1, "量程"=enum."低量程"} ("参数簇"), "启动参数"=w331, "启动模式"=w333, "量程"=w332) -> (w329:T22)
    n245 = while {
      tunnel: w335 -> [w461]
      tunnel: w329 -> [w460]
      shift-right: [w455] -> _
      shift-left: _ -> [w457]
      shift-right: [w456] -> _
      shift-left: _ -> [w458]
      shift-right: ["流程路径"] -> _
      shift-left: _ -> [w453]
      stop <- TRUE stop-if-true
      n246 = Not Equal?(x=w453, y="流程路径") -> (x != y?=w451:bool)
      n247 = Or(x=w461, y=w451) -> (x .or. y?=w452:bool)
      n248 = case shown="真" w452 {
        tunnel: [w463 w471] -> w456
        tunnel: [w462 w470] -> w455
        tunnel: w460 -> [_ w465]
        tunnel: w458 -> [w463 _]
        tunnel: w457 -> [w462 _]
        tunnel: "流程路径" -> [_ w464]
        frame False {
        }
        frame True {
          n249 = call "斯坦道XML解析.vi"("添加的路径"=w464, "参数簇"=w465) -> ("步骤时间"=w466:string[], "步骤名"=w468:string[])  [unwired: 8 in]
          n250 = Build Array(w468, w466) -> (w467:string[][])
          n251 = for {
            tunnel: w468 -> [_] mode=indexing
            tunnel: [w472] -> w469 mode=indexing
            i -> [w472]
          }
          n252 = Transpose 2D Array(2D array=w467) -> (transposed array=w470:string[][])
          n253 = Number To Decimal String(number=w469) -> (decimal integer string=w471:string[])  [unwired: 1 in]
        }
      }
      n254 = property on="多列列表框" class="MCListbox (严格)"("ItemNames"=w455, "RowHdrs[]"=w456) -> ()  [unwired: 2 in, 2 out]
    }
    n255 = Wait (ms)(milliseconds to wait=u32 1000 ("等待时间（毫秒）")) -> ()  [unwired: 1 out]
  }
  n256 = Bundle("参数下拉列表"=w5, "测量模式下拉列表"=w4, "量程下拉列表"=w3) -> (w6:T25)  [unwired: 1 in]
  n257 = property on="曲线模型" class="曲线模型 (严格)"("属性"=w6) -> (error out=w7:errorcluster)  [unwired: 2 in, 1 out]
  n258 = control-ref of="量程参数读取"() -> (w12:refnum<vi>)
  n259 = control-ref of="公式"() -> (w13:refnum<vi>)
  n260 = control-ref of="参数下拉列表"() -> (w15:refnum<vi>)
  n261 = control-ref of="测量模式下拉列表"() -> (w14:refnum<vi>)
  n262 = control-ref of="量程下拉列表"() -> (w16:refnum<vi>)
  n263 = Obtain Queue(name (unnamed)="TP" ("名称（未命名）"), element data type=cluster{"命令":string, "data":variant} {"命令"="", "data"=variant}) -> (queue out=w18:refnum<queue>, error out=w19:errorcluster)  [unwired: 3 in, 1 out]
  n264 = while {
    tunnel: w18 -> [w490]
    tunnel: w19 -> [_]
    shift-right: [w488] -> _
    shift-left: enum16{"总磷", "总氮"}."总磷" ("枚举") -> [w489]
    stop <- FALSE stop-if-true
    n265 = global read "总磷总氮断电保存全局变量.vi" "流程路径"() -> (w487:path)
    n266 = global read "总磷总氮断电保存全局变量.vi" "VISA Resource"() -> (→"字符串 2":refnum<visa-resource-name>)
    n267 = Get Queue Status(queue=w490) -> (queue out=w485:refnum<queue>, # elements in queue=w484:i32)  [unwired: 2 in, 6 out]
    n268 = local write "流程路径"(w487) -> ()
    n269 = case shown="0" w484 {
      tunnel: w485 -> [_ w510]
      tunnel: w489 -> [w493 w507]
      tunnel: [w493 w505] -> w488
      frame Default {
      }
      frame 0 {
        # "试剂填充 172 \n管路清洗108\n氨氮92\n总磷131\n总磷海水147\n总氮76\n总氮海水92"
        n270 = case shown="\"总氮\", 默认" w507 {
          selector: w507 -> [w524 w526]
          tunnel: [w525 w527] -> w508
          tunnel: [w524 w526] -> w506
          frame "总氮", Default {
            w525 = u16 2 items=["总磷"=1, "总氮"=2] ("站号")
          }
          frame "总磷" {
            w527 = u16 1 items=["总磷"=1, "氨氮"=3] ("站号")
          }
        }
        n271 = global read "VAR总磷总氮全局变量.vi" "状态告警区"() -> (w497:T7)
        n272 = Unbundle By Name(w497) -> ("系统时间"=w504:timestamp, "工作状态"=w496:T8)
        n273 = Get Date/Time In Seconds() -> (seconds since 1Jan1904=w503:timestamp)
        n274 = Equal?(x=w496, y=T8."空闲") -> (x = y?=w494:bool)
        n275 = Subtract(x=w503, y=w504) -> (x-y=w502:dbl)
        n276 = Bundle By Name(cluster=cluster{"命令":string, "data":variant} {"命令"="", "data"=variant} ("元素"), "命令"="读状态告警区", "data"=w508) -> (w512:cluster{"命令":string, "data":variant})
        n277 = Absolute Value(x=w502) -> (abs(x)=w501:dbl)
        n278 = Enqueue Element(queue=w510, element=w512) -> (queue out=w509:refnum<queue>)  [unwired: 2 in, 2 out]
        n279 = case shown="真" w494 {
          tunnel: w509 -> [w514 w517]
          tunnel: w508 -> [_ w516]
          tunnel: [w514 w515] -> w498
          frame False {
          }
          frame True {
            n280 = Bundle By Name(cluster=cluster{"命令":string, "data":variant} {"命令"="", "data"=variant} ("元素"), "命令"="读测量数据区", "data"=w516) -> (w519:cluster{"命令":string, "data":variant})
            n281 = Enqueue Element(queue=w517, element=w519) -> (queue out=w515:refnum<queue>)  [unwired: 2 in, 2 out]
          }
        }
        n282 = Greater Or Equal?(x=w501, y=120.0) -> (x >= y?=w499:bool)
        n283 = Increment(x=w506) -> (x+1=w505:enum16{"总磷", "总氮"})
        n284 = case shown="真" w499 {
          tunnel: w498 -> [_ w522]
          frame False {
          }
          frame True {
            n285 = call "总磷总氮启动命令.vi"("参数"=T26 {"站号"=3, "量程切换"=enum."AUTO", "控制命令"=enum."校时", "模式设置"=enum."待机", "测量间隔"=0}) -> ("启动命令"=w521:cluster{"命令":string, "data":variant})  [unwired: 10 in]
            n286 = Enqueue Element(queue=w522, element=w521) -> ()  [unwired: 2 in, 3 out]
          }
        }
      }
    }
    n287 = Wait (ms)(milliseconds to wait=u32 1000 ("等待时间（毫秒）")) -> ()  [unwired: 1 out]
  }
  n288 = while {
    tunnel: w18 -> [w533]
    tunnel: w16 -> [w532]
    tunnel: w15 -> [w531]
    tunnel: w14 -> [w530]
    tunnel: w13 -> [w529]
    tunnel: w12 -> [w528]
    tunnel: w7 -> [_]
    stop <- FALSE stop-if-true
    n289 = event shown="[14] \"单步测试\": 值改变" {
      selector: _ -> [_ _ _ _ _ _ _ _ _ _ _ _ _ _ _ _ _ _ _ _ _ _ _]
      dyn-events: _ -> [_ _ _ _ _ _ _ _ _ _ _ _ _ _ _ _ _ _ _ _ _ _ _]
      timeout: _ -> [_ _ _ _ _ _ _ _ _ _ _ _ _ _ _ _ _ _ _ _ _ _ _]
      tunnel: w533 -> [_ _ _ _ w553 w581 _ _ _ _ _ _ _ w726 _ w732 _ _ _ _ _ _ _]
      tunnel: w532 -> [_ _ _ _ _ _ _ _ _ _ _ _ _ _ _ _ _ _ _ w748 _ _ _]
      tunnel: w531 -> [_ _ _ _ _ _ _ _ _ _ _ _ _ _ _ _ _ _ _ w746 _ w787 w794]
      tunnel: w530 -> [_ _ _ _ _ _ _ _ _ _ _ _ _ _ _ _ _ _ _ w747 _ _ _]
      tunnel: w529 -> [_ _ _ _ _ _ _ _ _ _ _ _ _ _ _ _ _ _ _ w742 _ _ _]
      tunnel: w528 -> [_ _ _ _ _ _ _ _ _ _ _ _ _ _ _ _ _ _ _ _ _ w785 _]
      tunnel: [_ _ w539 _ _ _ _ _ _ _ _ _ _ _ _ _ _ _ _ _ _ _ _] -> _
      event Timeout {
        n290 = event-data() -> ()  [unwired: 1 in, 3 out]
      }
      event "布尔": Mouse Down {
        n291 = event-data() -> ("CtlRef"=w536:refnum<vi>)  [unwired: 1 in, 5 out]
        n292 = property class="Bool (严格)"(reference=w536) -> ("Value"=w535:bool)  [unwired: 1 in, 2 out]
        n293 = case shown="真" w535 {
          frame False {
            n294 = call "密码键盘.vi"() -> ("NewNumber"=→"输入密码":dbl)  [unwired: 1 in]
          }
          frame True {
            n295 = local write "输入密码"(u32 0 ("输入密码")) -> ()
          }
        }
      }
      event "测量模式下拉列表", "量程下拉列表", "参数下拉列表": Value Change {
        n296 = event-data() -> ()  [unwired: 1 in, 6 out]
        n297 = local read "参数下拉列表"() -> (w541:enum16{"总磷", "总氮"})
        n298 = local read "测量模式下拉列表"() -> (w542:enum16{"水样测量", "零点核查", "跨度核查", "标样核查", "加标回收"})
        n299 = local read "量程下拉列表"() -> (w543:enum16{"低量程", "高量程"})
        n300 = Bundle("参数下拉列表"=w541, "测量模式下拉列表"=w542, "量程下拉列表"=w543) -> (w540:T25)  [unwired: 1 in]
        n301 = property on="曲线模型" class="曲线模型 (严格)"("属性"=w540) -> (error out=w539:errorcluster)  [unwired: 2 in, 1 out]
      }
      event "流程固件": Value Change {
        n302 = event-data() -> ()  [unwired: 1 in, 6 out]
        n303 = call "流程固件设置对话框.vi"() -> ()  [unwired: 12 in]
      }
      event "串口设置": Value Change {
        n304 = event-data() -> ()  [unwired: 1 in, 6 out]
        n305 = global read "总磷总氮断电保存全局变量.vi" "VISA Resource"() -> (w550:refnum<visa-resource-name>)
        n306 = global read "总磷总氮断电保存全局变量.vi" "MB通信方式选择"() -> (w544:enum16{"串口", "TCP"})
        n307 = global read "总磷总氮断电保存全局变量.vi" "IP"() -> (w549:string)
        n308 = global read "总磷总氮断电保存全局变量.vi" "PORT"() -> (w548:string)
        n309 = call "串口配置.vi"("PORT"=w548, "IP"=w549, "MB通信方式选择"=w544, "请选择串口:"=w550) -> ("PORT 2"=w546:string, "IP 2"=w547:string, "确认 2"=w551:bool, "VISA资源名称 2"=w552:refnum<visa-resource-name>, "MB通信方式选择 2"=w545:enum16{"串口", "TCP"})  [unwired: 3 in]
        n310 = case shown="真" w551 {
          tunnel: w552 -> [_ w558]
          tunnel: w553 -> [_ w557]
          tunnel: w547 -> [_ w556]
          tunnel: w546 -> [_ w555]
          tunnel: w545 -> [_ w554]
          frame False {
          }
          frame True {
            n311 = flat-sequence {
              tunnel: w558 -> [w563]
              tunnel: w557 -> [w564]
              tunnel: w556 -> [w562]
              tunnel: w555 -> [w561]
              tunnel: w554 -> [w560]
              frame #0 {
                n312 = global write "总磷总氮断电保存全局变量.vi" "IP"(w562) -> ()
                n313 = global write "总磷总氮断电保存全局变量.vi" "PORT"(w561) -> ()
                n314 = global write "总磷总氮断电保存全局变量.vi" "MB通信方式选择"(w560) -> ()
                n315 = global write "总磷总氮断电保存全局变量.vi" "VISA Resource"(w563) -> ()
                n316 = Flush Queue(queue=w564) -> (queue out=w559:refnum<queue>)  [unwired: 1 in, 2 out]
                n317 = Enqueue Element(queue=w559, element=cluster{"命令":string, "data":variant} {"命令"="启用模块", "data"=variant} ("元素")) -> ()  [unwired: 2 in, 3 out]
              }
              frame #1 {
                n318 = call <vilib>:"Application Directory.vi"() -> ("Application Directory"=w579:path)
                n319 = Build Path(base path=w579, name or relative path="data\\sys.ini" ("名称或相对路径")) -> (appended path=w577:path)
                n320 = call <vilib>:"Open Config Data.vi"("configuration file path"=w577) -> ("error out"=w573:errorcluster, "refnum"=w576:T15)  [unwired: 8 in, 1 out]
                n321 = vi-ref "总磷总氮断电保存全局变量.vi"() -> (w575:refnum<vi>)
                n322 = call <userlib>:"Write Panel to INI__ogtk.vi"("error in (no error)"=w573, "VI ref"=w575, "refnum"=w576) -> ("error out"=w572:errorcluster, "refnum out"=w574:T15)  [unwired: 7 in]
                n323 = call <vilib>:"Close Config Data.vi"("error in (no error)"=w572, "refnum"=w574) -> ("error out"=w567:errorcluster, "file path"=w566:path)  [unwired: 8 in]
                n324 = Open/Create/Replace File(file path (use dialog)=w566, error in=w567) -> (refnum out=w570:refnum<file>, error out=w571:errorcluster)  [unwired: 4 in, 1 out]
                n325 = Flush File(refnum=w570, error in=w571) -> (refnum out=w569:refnum<file>, error out=w568:errorcluster)
                n326 = Close File(refnum=w569, error in=w568) -> ()  [unwired: 2 out]
              }
            }
          }
        }
      }
      event "模块启用": Value Change {
        n327 = event-data() -> ("OldVal"=w582:bool)  [unwired: 1 in, 5 out]
        n328 = Flush Queue(queue=w581) -> (queue out=w580:refnum<queue>)  [unwired: 1 in, 2 out]
        n329 = case shown="假" w582 {
          tunnel: w580 -> [w583 w585]
          frame False {
            n330 = Enqueue Element(queue=w583, element=cluster{"命令":string, "data":variant} {"命令"="停用模块", "data"=variant} ("元素")) -> ()  [unwired: 2 in, 3 out]
          }
          frame True {
            n331 = Enqueue Element(queue=w585, element=cluster{"命令":string, "data":variant} {"命令"="启用模块", "data"=variant} ("元素")) -> ()  [unwired: 2 in, 3 out]
          }
        }
      }
      event "流程路径": Value Change {
        n332 = event-data() -> ()  [unwired: 1 in, 6 out]
        n333 = flat-sequence {
          frame #0 {
            n334 = local read "流程路径"() -> (w587:path)
            n335 = global write "总磷总氮断电保存全局变量.vi" "流程路径"(w587) -> ()
          }
          frame #1 {
            n336 = call <vilib>:"Application Directory.vi"() -> ("Application Directory"=w601:path)
            n337 = Build Path(base path=w601, name or relative path="data\\sys.ini" ("名称或相对路径")) -> (appended path=w599:path)
            n338 = call <vilib>:"Open Config Data.vi"("configuration file path"=w599) -> ("error out"=w595:errorcluster, "refnum"=w598:T15)  [unwired: 8 in, 1 out]
            n339 = vi-ref "总磷总氮断电保存全局变量.vi"() -> (w597:refnum<vi>)
            n340 = call <userlib>:"Write Panel to INI__ogtk.vi"("error in (no error)"=w595, "VI ref"=w597, "refnum"=w598) -> ("error out"=w594:errorcluster, "refnum out"=w596:T15)  [unwired: 7 in]
            n341 = call <vilib>:"Close Config Data.vi"("error in (no error)"=w594, "refnum"=w596) -> ("error out"=w589:errorcluster, "file path"=w588:path)  [unwired: 8 in]
            n342 = Open/Create/Replace File(file path (use dialog)=w588, error in=w589) -> (refnum out=w592:refnum<file>, error out=w593:errorcluster)  [unwired: 4 in, 1 out]
            n343 = Flush File(refnum=w592, error in=w593) -> (refnum out=w591:refnum<file>, error out=w590:errorcluster)
            n344 = Close File(refnum=w591, error in=w590) -> ()  [unwired: 2 out]
          }
        }
      }
      event "公式一键写入": Value Change {
        n345 = event-data() -> ()  [unwired: 1 in, 6 out]
        n346 = local read "公式"() -> (w602:cluster{"X^2":dbl, "X":dbl, "b":dbl})
        n347 = call "公式复合写入.vi"("公式"=w602) -> ()  [unwired: 11 in]
      }
      event "曲线模型": Value Change {
        n348 = event-data() -> ()  [unwired: 1 in, 6 out]
        n349 = Unbundle By Name("曲线模型") -> ("X^2"=w606:dbl, "X"=w605:dbl, "B"=w604:dbl)
        n350 = Bundle("X^2"=w606, "X"=w605, "B"=w604) -> (w603:cluster{"X^2":dbl, "X":dbl, "B":dbl})  [unwired: 1 in]
        n351 = local write "公式"(w603) -> ()
      }
      event "质控参数设置": Value Change {
        n352 = event-data() -> ()  [unwired: 1 in, 6 out]
        n353 = global read "总磷总氮断电保存全局变量.vi" "质控参数设置"() -> (w608:T27)
        n354 = call "总磷总氮质控参数设置.vi"("质控参数设置"=w608) -> ("输出簇"=w609:T28)  [unwired: 10 in]
        n355 = Unbundle By Name(w609) -> ("确定"=w610:bool)
        n356 = case shown="真" w610 {
          tunnel: w609 -> [_ w612]
          tunnel: w608 -> [_ w611]
          frame False {
          }
          frame True {
            n357 = flat-sequence {
              tunnel: w612 -> [w623]
              tunnel: w611 -> [w622]
              frame #0 {
                n358 = Unbundle By Name(w623) -> ("总磷跨度值"=w621:dbl, "总磷零点标准液浓度"=w620:dbl, "总磷跨度标准液浓度"=w619:dbl, "总磷标准液标准浓度"=w618:dbl, "总氮跨度值"=w617:dbl, "总氮零点标准液浓度"=w616:dbl, "总氮跨度标准液浓度"=w615:dbl, "总氮标准液标准浓度"=w614:dbl)
                n359 = Bundle By Name(cluster=w622, "总磷跨度值"=w621, "总磷零点标准液浓度"=w620, "总磷跨度标准液浓度"=w619, "总磷标准液标准浓度"=w618, "总氮跨度值"=w617, "总氮零点标准液浓度"=w616, "总氮跨度标准液浓度"=w615, "总氮标准液标准浓度"=w614) -> (w613:T27)
                n360 = global write "总磷总氮断电保存全局变量.vi" "质控参数设置"(w613) -> ()
              }
              frame #1 {
                n361 = call <vilib>:"Application Directory.vi"() -> ("Application Directory"=w637:path)
                n362 = Build Path(base path=w637, name or relative path="data\\sys.ini" ("名称或相对路径")) -> (appended path=w635:path)
                n363 = call <vilib>:"Open Config Data.vi"("configuration file path"=w635) -> ("error out"=w631:errorcluster, "refnum"=w634:T15)  [unwired: 8 in, 1 out]
                n364 = vi-ref "总磷总氮断电保存全局变量.vi"() -> (w633:refnum<vi>)
                n365 = call <userlib>:"Write Panel to INI__ogtk.vi"("error in (no error)"=w631, "VI ref"=w633, "refnum"=w634) -> ("error out"=w630:errorcluster, "refnum out"=w632:T15)  [unwired: 7 in]
                n366 = call <vilib>:"Close Config Data.vi"("error in (no error)"=w630, "refnum"=w632) -> ("error out"=w625:errorcluster, "file path"=w624:path)  [unwired: 8 in]
                n367 = Open/Create/Replace File(file path (use dialog)=w624, error in=w625) -> (refnum out=w628:refnum<file>, error out=w629:errorcluster)  [unwired: 4 in, 1 out]
                n368 = Flush File(refnum=w628, error in=w629) -> (refnum out=w627:refnum<file>, error out=w626:errorcluster)
                n369 = Close File(refnum=w627, error in=w626) -> ()  [unwired: 2 out]
              }
            }
          }
        }
      }
      event "总氮参数设置": Value Change {
        n370 = event-data() -> ()  [unwired: 1 in, 6 out]
        n371 = global read "总磷总氮断电保存全局变量.vi" "总氮仪器参数"() -> (w639:T29)
        n372 = call "仪器参数设置.vi"("氨氮仪器参数"=w639) -> ("仪器参数设置输出"=w638:T30)  [unwired: 10 in]
        n373 = Unbundle By Name(w638) -> ("确定"=w640:bool)
        n374 = case shown="真" w640 {
          tunnel: w638 -> [_ w642]
          tunnel: w639 -> [_ w641]
          frame False {
          }
          frame True {
            n375 = flat-sequence {
              tunnel: w642 -> [w658]
              tunnel: w641 -> [w657]
              frame #0 {
                n376 = Unbundle By Name(w658) -> ("测量量程"=w656:dbl, "测量精度"=w655:dbl, "测量间隔"=w654:dbl, "消解温度"=w653:dbl, "消解时长"=w652:dbl, "空白校准时间"=w651:timestamp, "曲线截距"=w650:dbl, "曲线斜率"=w649:dbl, "测量检出限"=w647:dbl, "测量信号值"=w646:dbl, "线性相关系数"=w645:dbl, "二次多项式系数"=w644:dbl, "标样校准时间"=w643:timestamp)
                n377 = Bundle By Name(cluster=w657, "测量量程"=w656, "测量精度"=w655, "测量间隔"=w654, "消解温度"=w653, "消解时长"=w652, "空白校准时间"=w651, "曲线截距"=w650, "曲线斜率"=w649, "测量检出限"=w647, "测量信号值"=w646, "线性相关系数"=w645, "二次多项式系数"=w644, "标样校准时间"=w643) -> (w648:T29)
                n378 = global write "总磷总氮断电保存全局变量.vi" "总氮仪器参数"(w648) -> ()
              }
              frame #1 {
                n379 = call <vilib>:"Application Directory.vi"() -> ("Application Directory"=w672:path)
                n380 = Build Path(base path=w672, name or relative path="data\\sys.ini" ("名称或相对路径")) -> (appended path=w670:path)
                n381 = call <vilib>:"Open Config Data.vi"("configuration file path"=w670) -> ("error out"=w666:errorcluster, "refnum"=w669:T15)  [unwired: 8 in, 1 out]
                n382 = vi-ref "总磷总氮断电保存全局变量.vi"() -> (w668:refnum<vi>)
                n383 = call <userlib>:"Write Panel to INI__ogtk.vi"("error in (no error)"=w666, "VI ref"=w668, "refnum"=w669) -> ("error out"=w665:errorcluster, "refnum out"=w667:T15)  [unwired: 7 in]
                n384 = call <vilib>:"Close Config Data.vi"("error in (no error)"=w665, "refnum"=w667) -> ("error out"=w660:errorcluster, "file path"=w659:path)  [unwired: 8 in]
                n385 = Open/Create/Replace File(file path (use dialog)=w659, error in=w660) -> (refnum out=w663:refnum<file>, error out=w664:errorcluster)  [unwired: 4 in, 1 out]
                n386 = Flush File(refnum=w663, error in=w664) -> (refnum out=w662:refnum<file>, error out=w661:errorcluster)
                n387 = Close File(refnum=w662, error in=w661) -> ()  [unwired: 2 out]
              }
            }
          }
        }
      }
      event "总磷参数设置": Value Change {
        n388 = event-data() -> ()  [unwired: 1 in, 6 out]
        n389 = global read "总磷总氮断电保存全局变量.vi" "总磷仪器参数"() -> (w674:T29)
        n390 = call "仪器参数设置.vi"("氨氮仪器参数"=w674) -> ("仪器参数设置输出"=w673:T30)  [unwired: 10 in]
        n391 = Unbundle By Name(w673) -> ("确定"=w675:bool)
        n392 = case shown="真" w675 {
          tunnel: w673 -> [_ w677]
          tunnel: w674 -> [_ w676]
          frame False {
          }
          frame True {
            n393 = flat-sequence {
              tunnel: w677 -> [w693]
              tunnel: w676 -> [w692]
              frame #0 {
                n394 = Unbundle By Name(w693) -> ("测量量程"=w691:dbl, "测量精度"=w690:dbl, "测量间隔"=w689:dbl, "消解温度"=w688:dbl, "消解时长"=w687:dbl, "空白校准时间"=w686:timestamp, "曲线截距"=w685:dbl, "曲线斜率"=w684:dbl, "测量检出限"=w682:dbl, "测量信号值"=w681:dbl, "线性相关系数"=w680:dbl, "二次多项式系数"=w679:dbl, "标样校准时间"=w678:timestamp)
                n395 = Bundle By Name(cluster=w692, "测量量程"=w691, "测量精度"=w690, "测量间隔"=w689, "消解温度"=w688, "消解时长"=w687, "空白校准时间"=w686, "曲线截距"=w685, "曲线斜率"=w684, "测量检出限"=w682, "测量信号值"=w681, "线性相关系数"=w680, "二次多项式系数"=w679, "标样校准时间"=w678) -> (w683:T29)
                n396 = global write "总磷总氮断电保存全局变量.vi" "总磷仪器参数"(w683) -> ()
              }
              frame #1 {
                n397 = call <vilib>:"Application Directory.vi"() -> ("Application Directory"=w707:path)
                n398 = Build Path(base path=w707, name or relative path="data\\sys.ini" ("名称或相对路径")) -> (appended path=w705:path)
                n399 = call <vilib>:"Open Config Data.vi"("configuration file path"=w705) -> ("error out"=w701:errorcluster, "refnum"=w704:T15)  [unwired: 8 in, 1 out]
                n400 = vi-ref "总磷总氮断电保存全局变量.vi"() -> (w703:refnum<vi>)
                n401 = call <userlib>:"Write Panel to INI__ogtk.vi"("error in (no error)"=w701, "VI ref"=w703, "refnum"=w704) -> ("error out"=w700:errorcluster, "refnum out"=w702:T15)  [unwired: 7 in]
                n402 = call <vilib>:"Close Config Data.vi"("error in (no error)"=w700, "refnum"=w702) -> ("error out"=w695:errorcluster, "file path"=w694:path)  [unwired: 8 in]
                n403 = Open/Create/Replace File(file path (use dialog)=w694, error in=w695) -> (refnum out=w698:refnum<file>, error out=w699:errorcluster)  [unwired: 4 in, 1 out]
                n404 = Flush File(refnum=w698, error in=w699) -> (refnum out=w697:refnum<file>, error out=w696:errorcluster)
                n405 = Close File(refnum=w697, error in=w696) -> ()  [unwired: 2 out]
              }
            }
          }
        }
      }
      event "总磷自动测试量程配置", "总氮自动测试量程配置": Value Change {
        n406 = event-data() -> ()  [unwired: 1 in, 6 out]
        n407 = flat-sequence {
          frame #0 {
            n408 = global write "总磷总氮断电保存全局变量.vi" "总氮自动测试量程配置"("总氮自动测试量程配置") -> ()
            n409 = global write "总磷总氮断电保存全局变量.vi" "总磷自动测试量程配置"("总磷自动测试量程配置") -> ()
          }
          frame #1 {
            n410 = call <vilib>:"Application Directory.vi"() -> ("Application Directory"=w723:path)
            n411 = Build Path(base path=w723, name or relative path="data\\sys.ini" ("名称或相对路径")) -> (appended path=w721:path)
            n412 = call <vilib>:"Open Config Data.vi"("configuration file path"=w721) -> ("error out"=w717:errorcluster, "refnum"=w720:T15)  [unwired: 8 in, 1 out]
            n413 = vi-ref "总磷总氮断电保存全局变量.vi"() -> (w719:refnum<vi>)
            n414 = call <userlib>:"Write Panel to INI__ogtk.vi"("error in (no error)"=w717, "VI ref"=w719, "refnum"=w720) -> ("error out"=w716:errorcluster, "refnum out"=w718:T15)  [unwired: 7 in]
            n415 = call <vilib>:"Close Config Data.vi"("error in (no error)"=w716, "refnum"=w718) -> ("error out"=w711:errorcluster, "file path"=w710:path)  [unwired: 8 in]
            n416 = Open/Create/Replace File(file path (use dialog)=w710, error in=w711) -> (refnum out=w714:refnum<file>, error out=w715:errorcluster)  [unwired: 4 in, 1 out]
            n417 = Flush File(refnum=w714, error in=w715) -> (refnum out=w713:refnum<file>, error out=w712:errorcluster)
            n418 = Close File(refnum=w713, error in=w712) -> ()  [unwired: 2 out]
          }
        }
      }
      event "手动启动": Value Change {
        n419 = event-data() -> ()  [unwired: 1 in, 6 out]
        n420 = call "总磷总氮启动参数对话框.vi"() -> ("确认"=w724:bool, "元素"=w725:cluster{"命令":string, "data":variant})  [unwired: 10 in]
        n421 = case shown="真" w724 {
          tunnel: w726 -> [_ w728]
          tunnel: w725 -> [_ w727]
          frame False {
          }
          frame True {
            n422 = Enqueue Element(queue=w728, element=w727) -> ()  [unwired: 2 in, 3 out]
          }
        }
      }
      event "单步测试": Value Change {
        n423 = event-data() -> ()  [unwired: 1 in, 6 out]
        n424 = call "总磷单步调试对话框.vi"() -> ()  [unwired: 12 in]
      }
      event "停止": Value Change {
        n425 = event-data() -> ()  [unwired: 1 in, 6 out]
        n426 = Enqueue Element(queue=w732, element=cluster{"命令":string, "data":variant} {"命令"="启动", "data"=variant(cluster{"站号":u16, "控制命令输出":u16[]} {"站号"=1, "控制命令输出"=[2816]})} ("元素")) -> (queue out=w729:refnum<queue>)  [unwired: 2 in, 2 out]
        n427 = Enqueue Element(queue=w729, element=cluster{"命令":string, "data":variant} {"命令"="启动", "data"=variant(cluster{"站号":u16, "控制命令输出":u16[]} {"站号"=2, "控制命令输出"=[2816]})} ("元素")) -> ()  [unwired: 2 in, 3 out]
      }
      event "参数设置": Value Change {
        n428 = event-data() -> ()  [unwired: 1 in, 6 out]
        n429 = property on="窗格" class="Pane"("Origin"=T16 {"Horizontal"=0, "Vertical"=628} ("原点")) -> ()  [unwired: 2 in, 2 out]
      }
      event "返回": Value Change {
        n430 = event-data() -> ()  [unwired: 1 in, 6 out]
        n431 = property on="窗格" class="Pane"("Origin"=T16 {"Horizontal"=0, "Vertical"=0} ("原点")) -> ()  [unwired: 2 in, 2 out]
      }
      event "公式.X^2", "公式.X", "公式.b", "量程参数读取.测量精度", "量程参数读取.检出限", "量程参数读取.上限", "量程参数读取.下限", "量程参数读取.阈值（低->高）", "量程参数读取.阈值（高->低）", "量程参数读取.稀释度": Mouse Down {
        n432 = event-data() -> ("CtlRef"=w738:refnum<vi>)  [unwired: 1 in, 7 out]
        n433 = property class="DigNum (严格)"(reference=w738) -> (reference out=w736:refnum<vi>, "Value"=w737:dbl)  [unwired: 1 in, 1 out]
        n434 = call "数字键盘.vi"("OldNumber"=w737) -> ("NewNumber"=w735:dbl)
        n435 = property class="DigNum (严格)"(reference=w736, "Val(Sgnl)"=w735) -> ()  [unwired: 1 in, 2 out]
      }
      event "读公式": Value Change {
        n436 = event-data() -> ()  [unwired: 1 in, 6 out]
        n437 = property class="Enum (严格)"(reference=w746) -> ("Value"=w745:enum16{"总磷", "总氮"})  [unwired: 1 in, 2 out]
        n438 = property class="Enum (严格)"(reference=w747) -> ("Value"=w744:enum16{"水样测量", "零点核查", "跨度核查", "标样核查", "加标回收"})  [unwired: 1 in, 2 out]
        n439 = property class="Enum (严格)"(reference=w748) -> ("Value"=w743:enum16{"低量程", "高量程"})  [unwired: 1 in, 2 out]
        n440 = call "总磷总氮公式读取.vi"("量程"=w743, "测量模式"=w744, "测量参数"=w745) -> ("error out"=w740:errorcluster, "公式"=w741:cluster{"X^2":dbl, "X":dbl, "b":dbl})  [unwired: 7 in]
        n441 = property class="Clust (严格)"(reference=w742, "Value"=w741) -> ()  [unwired: 1 in, 2 out]
        n442 = case shown="错误" w740 {
          tunnel: ["读取成功" ("消息") "读取失败" ("消息")] -> w739
          frame No Error {
          }
          frame Error {
          }
        }
        n443 = One Button Dialog(message=w739) -> ()  [unwired: 1 in, 1 out]
      }
      event "写公式": Value Change {
        n444 = event-data() -> ()  [unwired: 1 in, 6 out]
        n445 = call "总磷总氮公式写入.vi"("公式"="公式", "量程"="量程下拉列表", "测量模式"="测量模式下拉列表", "测量参数"="参数下拉列表") -> ("error out"=w755:errorcluster)  [unwired: 7 in]
        n446 = case shown="无错误" w755 {
          tunnel: ["写入成功" ("消息") "写入失败" ("消息")] -> w756
          tunnel: "测量模式下拉列表" -> [w765 _]
          tunnel: "量程下拉列表" -> [w763 _]
          tunnel: "参数下拉列表" -> [w758 _]
          tunnel: "公式" -> [w757 _]
          frame No Error {
            n447 = Equal?(x=w765, y=enum16{"水样测量", "零点核查", "跨度核查", "标样核查", "加标回收"}."水样测量" ("测量模式下拉列表")) -> (x = y?=w761:bool)
            n448 = Equal?(x=w763, y=enum16{"低量程", "高量程"}."低量程" ("量程下拉列表")) -> (x = y?=w760:bool)
            n449 = And(x=w761, y=w760) -> (x .and. y?=w759:bool)
            n450 = case shown="真" w759 {
              tunnel: w758 -> [_ w768]
              tunnel: w757 -> [_ w767]
              frame False {
              }
              frame True {
                n451 = case shown="\"总磷\", 默认" w768 {
                  tunnel: w767 -> [w769 w775]
                  frame "总磷", Default {
                    n452 = Unbundle By Name(w769) -> ("X^2"=w772:dbl, "X"=w771:dbl, "b"=w770:dbl)
                    n453 = global read "总磷总氮断电保存全局变量.vi" "总磷仪器参数"() -> (w773:T29)
                    n454 = Bundle By Name(cluster=w773, "曲线截距"=w770, "曲线斜率"=w771, "二次多项式系数"=w772) -> (w774:T29)
                    n455 = global write "总磷总氮断电保存全局变量.vi" "总磷仪器参数"(w774) -> ()
                  }
                  frame "总氮" {
                    n456 = Unbundle By Name(w775) -> ("X^2"=w778:dbl, "X"=w777:dbl, "b"=w776:dbl)
                    n457 = global read "总磷总氮断电保存全局变量.vi" "总氮仪器参数"() -> (w779:T29)
                    n458 = Bundle By Name(cluster=w779, "曲线截距"=w776, "曲线斜率"=w777, "二次多项式系数"=w778) -> (w780:T29)
                    n459 = global write "总磷总氮断电保存全局变量.vi" "总氮仪器参数"(w780) -> ()
                  }
                }
              }
            }
          }
          frame Error {
          }
        }
        n460 = One Button Dialog(message=w756) -> ()  [unwired: 1 in, 1 out]
      }
      event "量程切换阈值读取": Value Change {
        n461 = event-data() -> ()  [unwired: 1 in, 6 out]
        n462 = property class="Enum (严格)"(reference=w787) -> ("Value"=w786:enum16{"总磷", "总氮"})  [unwired: 1 in, 2 out]
        n463 = call "总磷总氮量程读取.vi"("测量参数"=w786) -> ("error out"=w783:errorcluster, "量程参数读取"=w782:T31)  [unwired: 9 in]
        n464 = property class="Clust (严格)"(reference=w785, "Value"=w782) -> ()  [unwired: 1 in, 2 out]
        n465 = case shown="错误" w783 {
          tunnel: ["读取成功" ("消息") "读取失败" ("消息")] -> w784
          frame No Error {
          }
          frame Error {
          }
        }
        n466 = One Button Dialog(message=w784) -> ()  [unwired: 1 in, 1 out]
      }
      event "量程切换阈值写入": Value Change {
        n467 = event-data() -> ()  [unwired: 1 in, 6 out]
        n468 = property class="Enum (严格)"(reference=w794) -> ("Value"=w790:enum16{"总磷", "总氮"})  [unwired: 1 in, 2 out]
        n469 = call "总磷总氮量程写入.vi"("量程参数写入"="量程参数读取", "测量参数"=w790) -> ("error out"=w792:errorcluster)  [unwired: 8 in]
        n470 = case shown="无错误" w792 {
          tunnel: ["写入成功" ("消息") "写入失败" ("消息")] -> w793
          frame No Error {
          }
          frame Error {
          }
        }
        n471 = One Button Dialog(message=w793) -> ()  [unwired: 1 in, 1 out]
      }
    }
  }
